vi "Calibration Main.vi"(8 "error in (no error)":errorcluster, 11 "Pump Calibration Config in":T1={"Settings"={"Cycle Period"=500.0, "Ismatech"={"VISA resource name"="", "Simulated?"=TRUE, "Pump Number"=1.0, "Reverse?"=FALSE}, "Masterflex"={"VISA resource name"="", "Simulated?"=TRUE, "Pump Number"=1.0, "Reverse?"=FALSE}, "Bronkhorst M13 Flow Meter"={"VISA resource name"="", "Simulated?"=TRUE}, "PID 2 Parameters"={"Input Device"=enum."Default", "Output Device"=enum."Default"}, "Bronkhorst M14"={"VISA resource name"="", "Simulated?"=FALSE}, "Tacmina Settings"={"Analog DAQ Task"="", "Digital DAQ Task"=""}, "KNF SIMDOS Settings"={"VISA resource name"="", "Simulated?"=TRUE}, "VICI M50 Settings"={"VISA resource name"="", "Simulated?"=TRUE, "Pump Letter"="", "Reverse?"=FALSE}, "FLOM Settings"={"VISA resource name"="", "Simulated?"=TRUE, "Pump Number"=0.0}, "Calibration Limits"={"Minimum (ml/min)"=0.0, "Maximum (ml/min)"=0.0, "Steps"=0.0}, "SSI PR Settings"={"VISA resource name"="", "Simulated?"=FALSE}}, "Flowmeter Output"=0.0, "Density"=0.0, "FL Temp"=0.0, "Speed %"=0.0, "File Refnum"=refnum, "Pump On?"=enum."Not Initialized"} {"Settings"."Masterflex"."Pump Number" min=1.0 max=20.0 step=1.0; "Settings"."Ismatech"."Pump Number" min=1.0 max=20.0 step=1.0}) -> (0 "error out":errorcluster, 3 "Pump Calibration Config out":T1={"Settings"={"Cycle Period"=500.0, "Ismatech"={"VISA resource name"="", "Simulated?"=TRUE, "Pump Number"=1.0, "Reverse?"=FALSE}, "Masterflex"={"VISA resource name"="", "Simulated?"=TRUE, "Pump Number"=1.0, "Reverse?"=FALSE}, "Bronkhorst M13 Flow Meter"={"VISA resource name"="", "Simulated?"=TRUE}, "PID 2 Parameters"={"Input Device"=enum."Default", "Output Device"=enum."Default"}, "Bronkhorst M14"={"VISA resource name"="", "Simulated?"=FALSE}, "Tacmina Settings"={"Analog DAQ Task"="", "Digital DAQ Task"=""}, "KNF SIMDOS Settings"={"VISA resource name"="", "Simulated?"=TRUE}, "VICI M50 Settings"={"VISA resource name"="", "Simulated?"=TRUE, "Pump Letter"="", "Reverse?"=FALSE}, "FLOM Settings"={"VISA resource name"="", "Simulated?"=TRUE, "Pump Number"=0.0}, "Calibration Limits"={"Minimum (ml/min)"=0.0, "Maximum (ml/min)"=0.0, "Steps"=0.0}, "SSI PR Settings"={"VISA resource name"="", "Simulated?"=FALSE}}, "Flowmeter Output"=0.0, "Density"=0.0, "FL Temp"=0.0, "Speed %"=0.0, "File Refnum"=refnum, "Pump On?"=enum."Not Initialized"} {"Settings"."Masterflex"."Pump Number" min=1.0 max=20.0 step=1.0; "Settings"."Ismatech"."Pump Number" min=1.0 max=20.0 step=1.0})   [LabVIEW 2018, in "Calibration.lvlib"]
uses:
  Pfizer Timed Seq/Software/Calibration VIs/Calibration.lvlib
  Pump Calibration Config.ctl
  Pfizer Timed Seq/Software/Ismatec ISM 831C/Controls/Ismatech Settings Cluster.ctl
  Pfizer Timed Seq/Software/Masterflex 7550-30/Controls/Settings Cluster.ctl
  Pfizer Timed Seq/Software/Bronkhorst M13 Flow Meter/Settings Cluster.ctl
  Pfizer Timed Seq/Software/Measure Instrument/PID Input Enum.ctl
  Pfizer Timed Seq/Software/Measure Instrument/PID 2 Output Enum.ctl
  Pfizer Timed Seq/Software/Mettler Toledo/Controls/Settings Cluster.ctl
  Pfizer Timed Seq/Software/Tacmina QI/Tacmina QI DAQ Setting.ctl
  Pfizer Timed Seq/Software/KNF Pump/Settings Cluster plus SIMDOS.ctl
  Pfizer Timed Seq/Software/VICI M50 Party Mode/Settings Cluster.ctl
  Pfizer Timed Seq/Software/FLOM Pump/Settings Cluster.ctl
  Pfizer Timed Seq/Software/SSI PR Class/SSI PR or LD Settings Cluster.ctl
  Pfizer Timed Seq/Software/Bronkhorst M14 Flow Meter/Settings Cluster.ctl
  Pfizer Timed Seq/Software/ASIA Pump/Pump Settings.ctl
  Pfizer Timed Seq/Software/Masterflex 75211/Masterflex 75211 DAQ Setting.ctl
  <vilib>/Platform/TimedLoop/XDataNode/timing_clust.ctl
  <vilib>/Platform/TimedLoop/XDataNode/nitl_modes.ctl
  <vilib>/Platform/TimedLoop/XDataNode/wakeup.ctl
  Pfizer Timed Seq/Software/support/Message Queue/Enqueue Message (Single).vi
  <vilib>/Utility/file.llb/Read Delimited Spreadsheet (string).vi
  <vilib>/Utility/file.llb/Write Delimited Spreadsheet (string).vi
  <vilib>/Platform/TimedLoop/XDataNode/XDataNode.xnode
  <vilib>/regexp/Match Regular Expression.xnode
  Pfizer Timed Seq/Software/KNF Pump/KNF SIMDOS.lvlib
  Pfizer Timed Seq/Software/Ismatec ISM 831C/Ismatec ISM 831C.lvlib
  Pfizer Timed Seq/Software/VICI M50 Party Mode/VICI M6 M50 Party Mode.lvlib
  Pfizer Timed Seq/Software/Masterflex 7550-30/Masterflex 7550-30.lvlib
  Pfizer Timed Seq/Software/FLOM Pump/FLOM Pump.lvlib
  Pfizer Timed Seq/Software/Bronkhorst M13 Flow Meter/Bronkhorst M13 Flow Meter.lvlib
  Pfizer Timed Seq/Software/Bronkhorst M14 Flow Meter/Bronkhorst M14 Flow Meter.lvlib
  Pfizer Timed Seq/Software/support/Message Queue/Message Queue.lvlib
  Pfizer Timed Seq/Software/SSI PR Class/SSI PR or LD Pump.lvlib
  Support/Engine.lvlib
  <vilib>/Analysis/NI_AALPro.lvlib
  <vilib>/Platform/TimedLoop/XDataNode/XDNodeRunTimeDep.lvlib
  Pfizer Timed Seq/Software/Mettler Toledo/Mettler Toledo.lvlib
  Pfizer Timed Seq/Software/Tacmina QI/Tacmina QI.lvlib
  Pfizer Timed Seq/Software/ASIA Pump.lvlib
  Pfizer Timed Seq/Software/Masterflex 75211/Masterflex 75211.lvlib
panel:
  out "Y array":dbl[](array[numeric])
  out "X array":dbl[](array[numeric])
  out "Output Selected":bool
  out "Input Selected":bool
  out "Step Array":dbl[](array[numeric])
  in  "?":enum32{"Settings", "Results"}(tab)
  in  "Settings Dialog":T16={"Cycle Period"=500.0, "Ismatech"={"VISA resource name"="", "Simulated?"=FALSE, "Pump Number"=1.0, "Reverse?"=FALSE}, "Masterflex"={"VISA resource name"="", "Simulated?"=FALSE, "Pump Number"=1.0, "Reverse?"=FALSE}, "Mettler"={"VISA resource name"="", "Simulated?"=FALSE}, "Bronkhorst M13 Flow Meter"={"VISA resource name"="", "Simulated?"=FALSE}, "Setup Parameters"={"Input Device"=enum."Default", "Output Device"=enum."Default"}, "Bronkhorst M14 Settings"={"VISA resource name"="", "Simulated?"=FALSE}, "Tacmina Settings"={"Analog DAQ Task"="", "Digital DAQ Task"=""}, "KNF SIMDOS Settings"={"VISA resource name"="", "Simulated?"=FALSE}, "ASIA Pump C"={"ASIA Pump #"=-1, "channel"=-1, "Simulated"=FALSE}, "VICI M50 Settings"={"VISA resource name"="", "Simulated?"=FALSE, "Pump Letter"="", "Reverse?"=FALSE}, "FLOM Settings"={"VISA resource name"="", "Simulated?"=FALSE, "Pump Number"=1.0}, "Calibration Limits"={"Minimum (ml/min)"=0.0, "Maximum (ml/min)"=0.0, "Steps"=0.0}, "File Name"="", "SSI PR Settings"={"VISA resource name"="", "Simulated?"=FALSE}, "Masterflex 75211 Settings"={"Analog DAQ Task"="", "Digital DAQ Task"=""}} {"Calibration Limits"."Maximum (ml/min)" max=16.5; "ASIA Pump C"."channel" min=-1 max=1 step=1; "Masterflex"."Pump Number" min=1.0 max=20.0 step=1.0; "Ismatech"."Pump Number" min=1.0 max=20.0 step=1.0}
  in  "Start Button":bool
  in  "Cancel Button":bool
  out "Y Intercept":dbl
  in  "Accept Button":bool
  in  "Decline Button":bool
  out "Calibration Graph":cluster{dbl[], dbl[]}[](graph)
  out "Calibration Slope":dbl
  out "R^2 Value":dbl format="%#.4g"
  out "Pump Status":enum16{"Off", "On", "Not Initialized"}(ring)
  # "Output Instruments"
  # "Input Instruments"
  # "Output Instruments"
  # "Input Instruments"
  # "Output Instruments"
  # "Input Instruments"
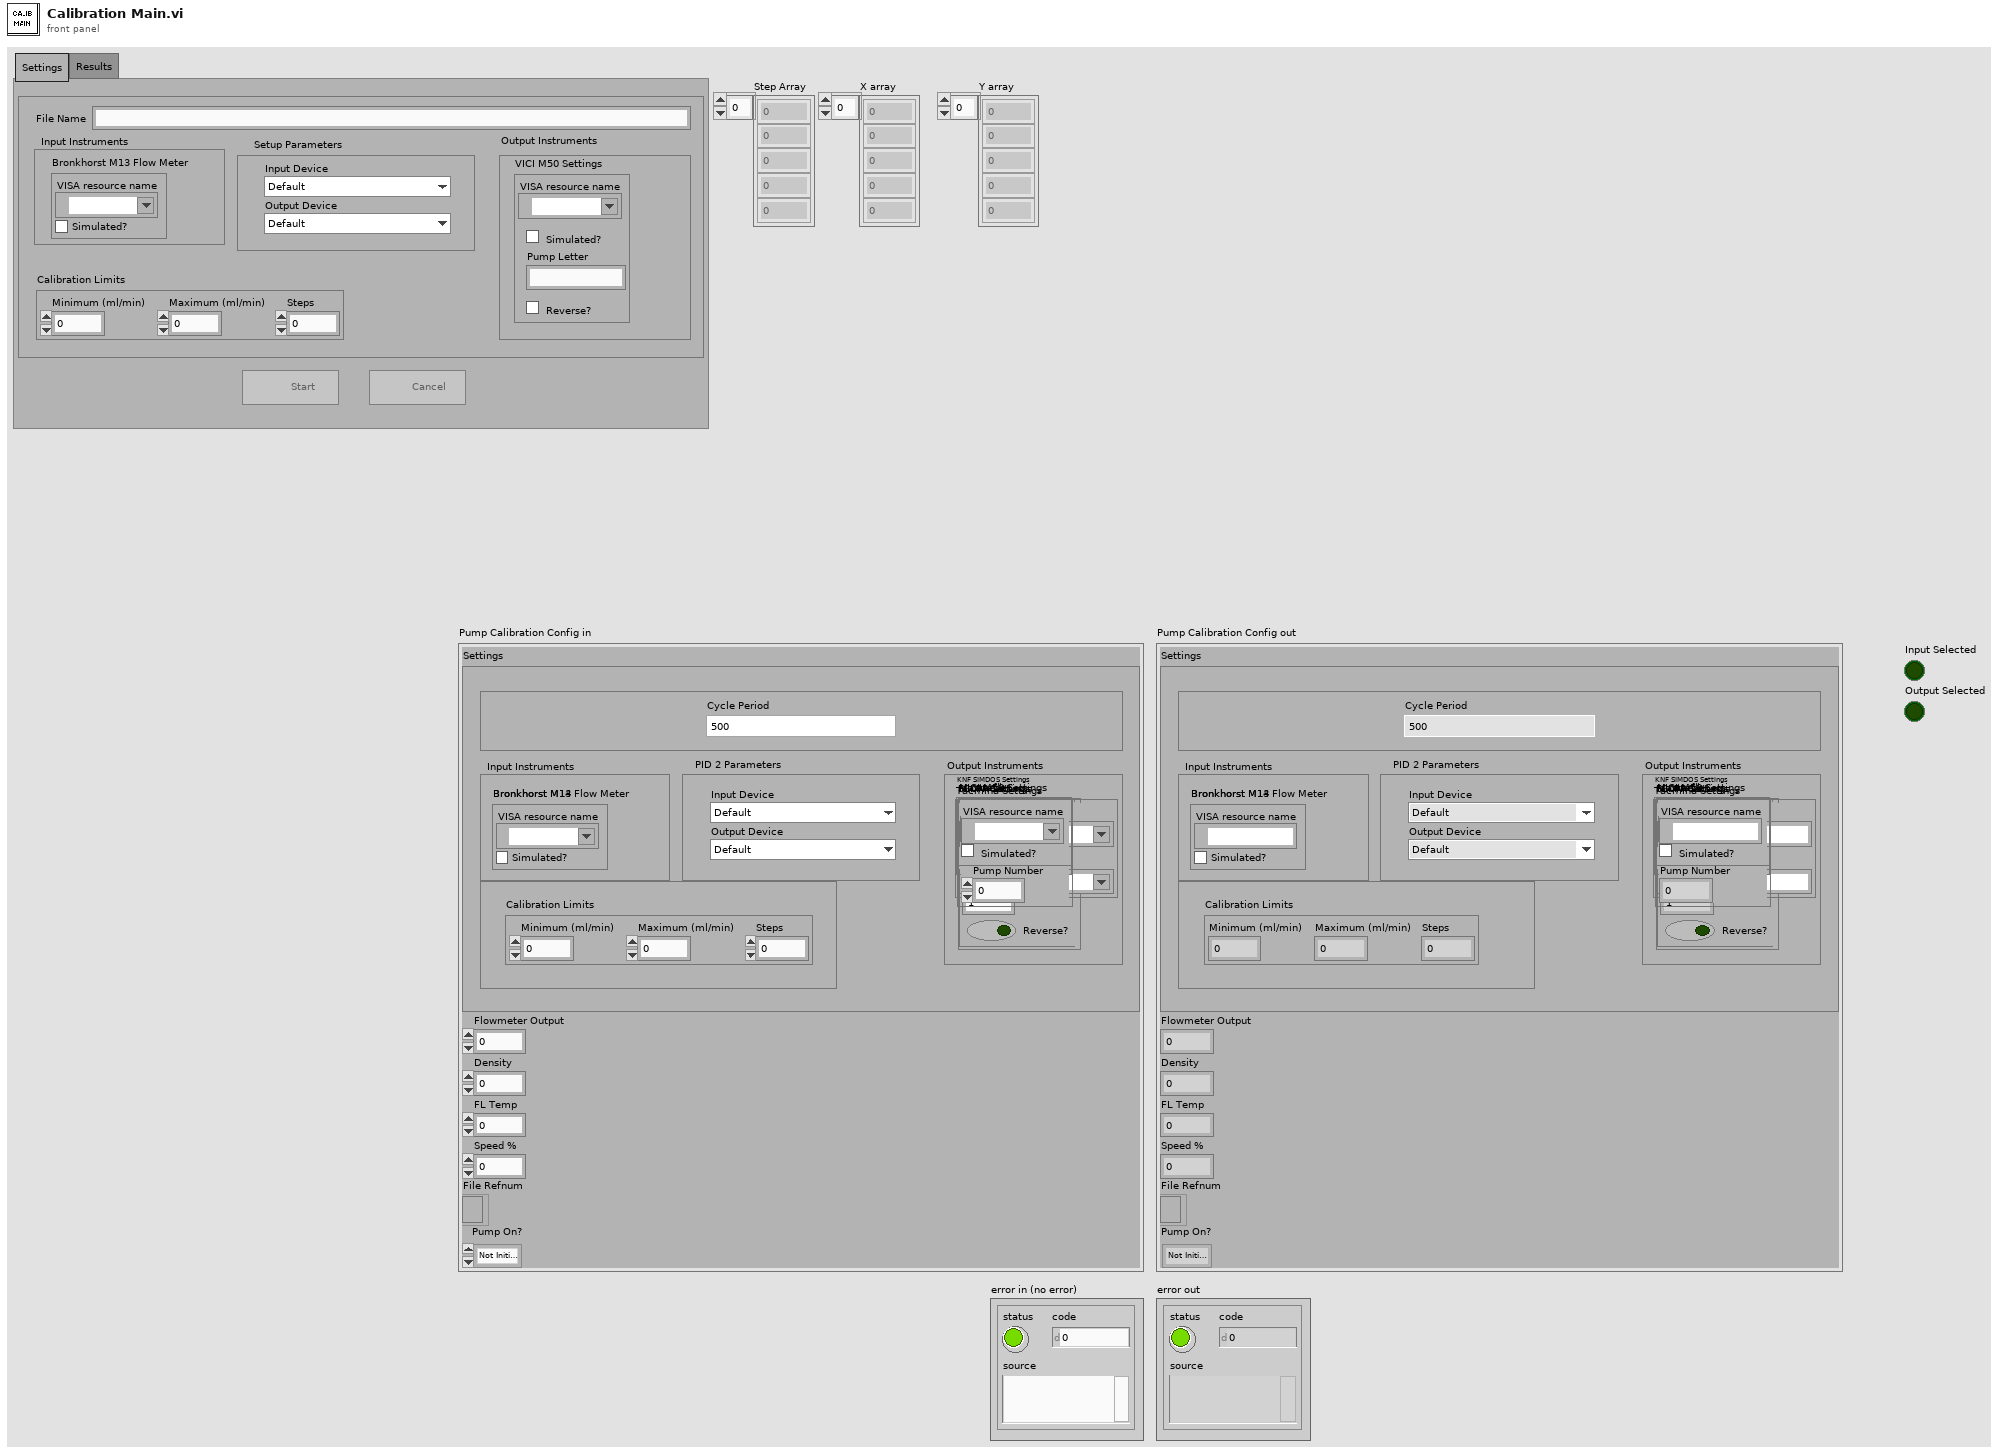
[diagram p1: front panel]
types:
  T1 = typedef "Calibration.lvlib/Pump Calibration Config.ctl" = cluster{"Settings":cluster{"Cycle Period":dbl, "Ismatech":T2, "Masterflex":T3, "Bronkhorst M13 Flow Meter":T4, "PID 2 Parameters":cluster{"Input Device":T5, "Output Device":T6}, "Bronkhorst M14":T7, "Tacmina Settings":T8, "KNF SIMDOS Settings":T9, "VICI M50 Settings":T10, "FLOM Settings":T11, "Calibration Limits":cluster{"Minimum (ml/min)":dbl, "Maximum (ml/min)":dbl, "Steps":dbl}, "SSI PR Settings":T12}, "Flowmeter Output":dbl, "Density":dbl, "FL Temp":dbl, "Speed %":dbl, "File Refnum":refnum<file>, "Pump On?":enum16{"Off", "On", "Not Initialized"}}
  T2 = typedef "Ismatec ISM 831C.lvlib/Ismatech Settings Cluster.ctl" = cluster{"VISA resource name":refnum<visa-resource-name>, "Simulated?":bool, "Pump Number":dbl, "Reverse?":bool}
  T3 = typedef "Masterflex 7550-30.lvlib/Settings Cluster.ctl" = cluster{"VISA resource name":refnum<visa-resource-name>, "Simulated?":bool, "Pump Number":dbl, "Reverse?":bool}
  T4 = typedef "Bronkhorst M13 Flow Meter.lvlib/Settings Cluster.ctl" = cluster{"VISA resource name":refnum<visa-resource-name>, "Simulated?":bool}
  T5 = typedef "PID Input Enum.ctl" = enum16{"Default", "Bronkhorst M13", "Bronkhorst M14", "Scale Rate of Change"}
  T6 = typedef "PID 2 Output Enum.ctl" = enum16{"Default", "Ismatec ISM 831C", "Masterflex 7550-30", "VICI", "Tacmina QI", "KNF SIMDOS", "ASIA Type C", "FLOM UI-22-11", "SSI PR/LD", "SSI P40", "Masterflex 75211-70"}
  T7 = typedef "Mettler Toledo.lvlib/Settings Cluster.ctl" = cluster{"VISA resource name":refnum<visa-resource-name>, "Simulated?":bool}
  T8 = typedef "Tacmina QI.lvlib/Tacmina QI DAQ Setting.ctl" = cluster{"Analog DAQ Task":refnum<k21>, "Digital DAQ Task":refnum<k21>}
  T9 = typedef "KNF SIMDOS.lvlib/Settings Cluster plus SIMDOS.ctl" = cluster{"VISA resource name":refnum<visa-resource-name>, "Simulated?":bool}
  T10 = typedef "VICI M6 M50 Party Mode.lvlib/Settings Cluster.ctl" = cluster{"VISA resource name":refnum<visa-resource-name>, "Simulated?":bool, "Pump Letter":string, "Reverse?":bool}
  T11 = typedef "FLOM Pump.lvlib/Settings Cluster.ctl" = cluster{"VISA resource name":refnum<visa-resource-name>, "Simulated?":bool, "Pump Number":dbl}
  T12 = typedef "SSI PR or LD Pump.lvlib/SSI PR or LD Settings Cluster.ctl" = cluster{"VISA resource name":refnum<visa-resource-name>, "Simulated?":bool}
  T13 = typedef "Bronkhorst M14 Flow Meter.lvlib/Settings Cluster.ctl" = cluster{"VISA resource name":refnum<visa-resource-name>, "Simulated?":bool}
  T14 = typedef "ASIA Pump.lvlib/Pump Settings.ctl" = cluster{"ASIA Pump #":i32, "channel":i32, "Simulated":bool}
  T15 = typedef "Masterflex 75211.lvlib/Masterflex 75211 DAQ Setting.ctl" = cluster{"Analog DAQ Task":refnum<k21>, "Digital DAQ Task":refnum<k21>}
  T16 = cluster{"Cycle Period":dbl, "Ismatech":T2, "Masterflex":T3, "Mettler":T7, "Bronkhorst M13 Flow Meter":T4, "Setup Parameters":cluster{"Input Device":T5, "Output Device":T6}, "Bronkhorst M14 Settings":T13, "Tacmina Settings":T8, "KNF SIMDOS Settings":T9, "ASIA Pump C":T14, "VICI M50 Settings":T10, "FLOM Settings":T11, "Calibration Limits":cluster{"Minimum (ml/min)":dbl, "Maximum (ml/min)":dbl, "Steps":dbl}, "File Name":string, "SSI PR Settings":T12, "Masterflex 75211 Settings":T15}
  T17 = enum8{"Enabled", "Disabled", "Disabled and Grayed Out"}
  T18 = cluster{"Calibration UI":refnum<queue>, "Calibration Engine":refnum<queue>}
  T19 = typedef "XDNodeRunTimeDep.lvlib/timing_clust.ctl" = cluster{"Expected End [f-1]":u64, "Actual End [f-1]":u64, "Finished Late? [f-1]":bool, "Expected End [i-1]":u64, "Actual End [i-1]":u64, "Finished Late? [i-1]":bool, "Expected Start [i]":u64, "Actual Start [i]":u64, "Expected Start [f]":u64, "Actual Start [f]":u64, "Source Name":string, "Structure Name":string, "Period":i64, "Deadline":i64, "Offset":i64, "Start":i64, "Priority":i32, "Timeout":i32, "Mode":T20, "Wakeup Reason":T21, "Error":errorcluster, "Source Type":string, "Secondary Source Type":string, "Global End Time":u64, "Global Start Time":u64, "Frame Duration":u64, "Iteration Duration":u64, "Assigned CPU":i32, "I/O Scan Engine Mode":u32}
  T20 = typedef "XDNodeRunTimeDep.lvlib/nitl_modes.ctl" = enum32{"No Change", "Process missed periods, maintain original phase", "Discard missed periods, maintain original phase", "Process missed periods, ignore original phase", "Discard missed periods, ignore original phase"}
  T21 = typedef "XDNodeRunTimeDep.lvlib/wakeup.ctl" = enum32{"Normal", "Aborted", "Asynchronous wakeup", "Timing source error", "Timed loop error", "Timeout"}
  T22 = enum16{"open", "replace", "create", "open or create", "replace or create", "replace or create with confirmation"}
  T23 = cluster{"slope min":dbl, "slope max":dbl, "intercept min":dbl, "intercept max":dbl}
  T24 = cluster{"Minimum (ml/min)":dbl, "Maximum (ml/min)":dbl, "Steps":dbl}
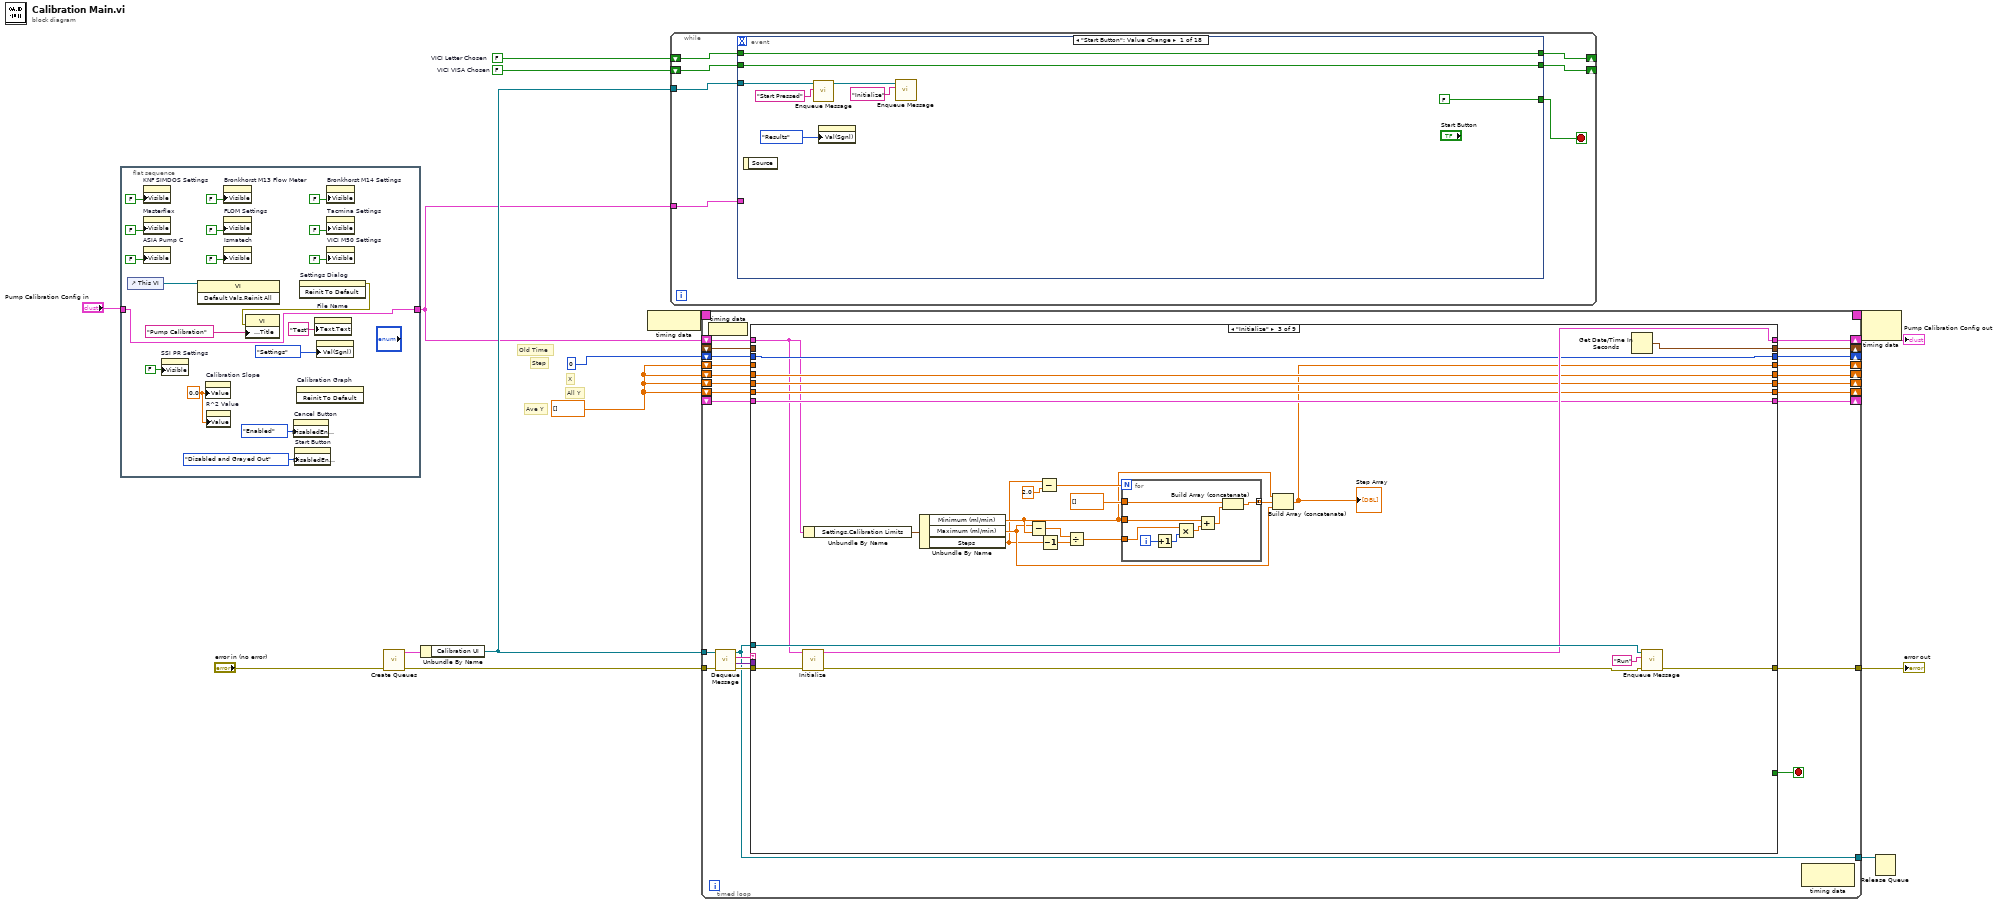
[diagram p0: block diagram]
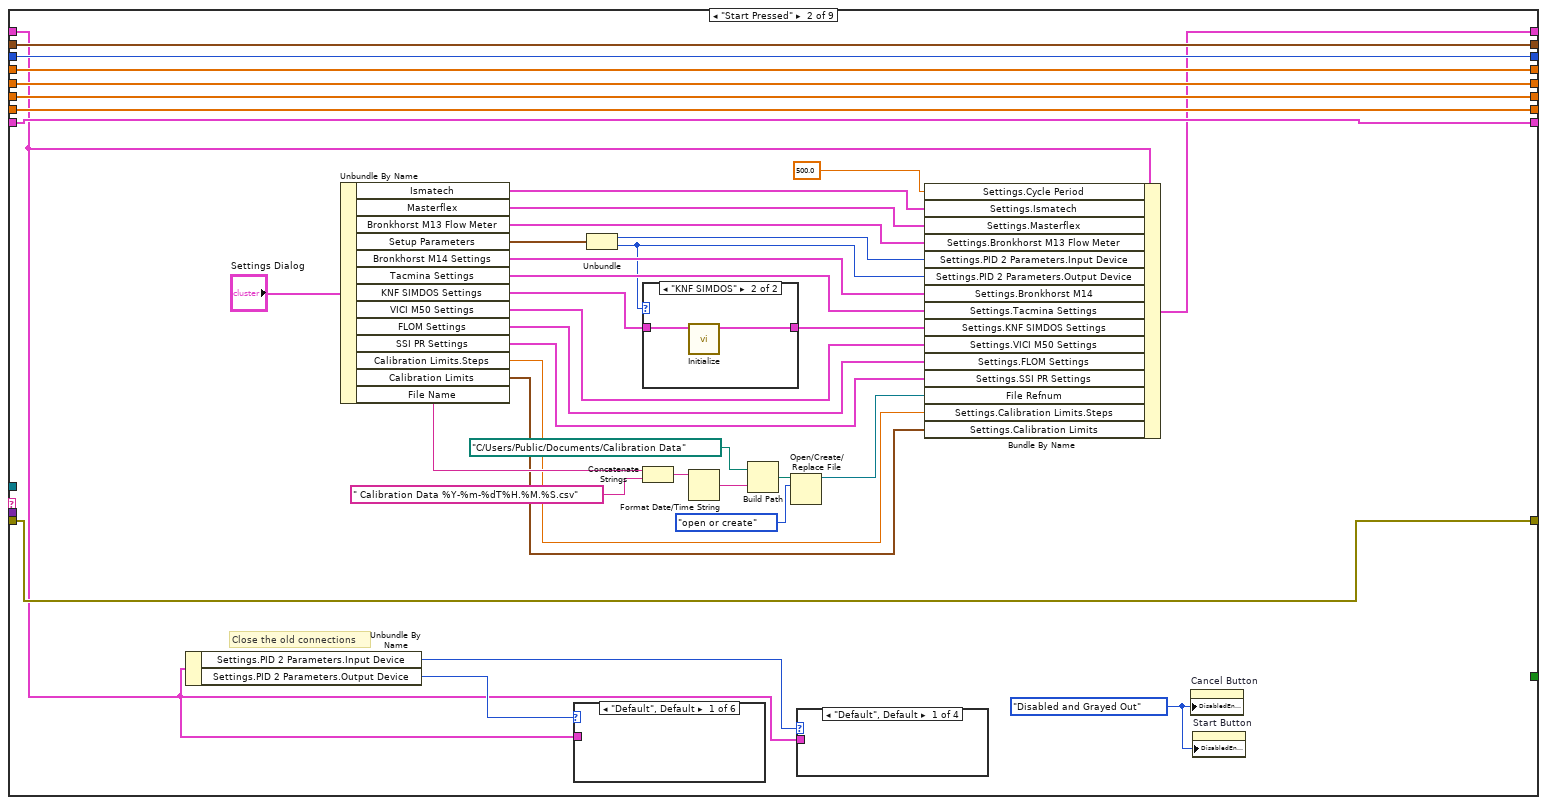
[diagram p3: hidden frame]
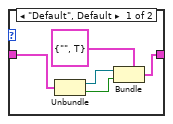
[diagram p4: hidden frame]
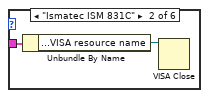
[diagram p5: hidden frame]
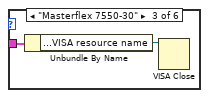
[diagram p6: hidden frame]
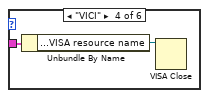
[diagram p7: hidden frame]
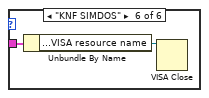
[diagram p9: hidden frame]
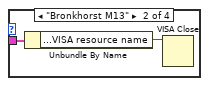
[diagram p10: hidden frame]
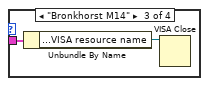
[diagram p11: hidden frame]
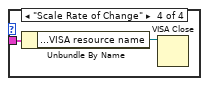
[diagram p12: hidden frame]
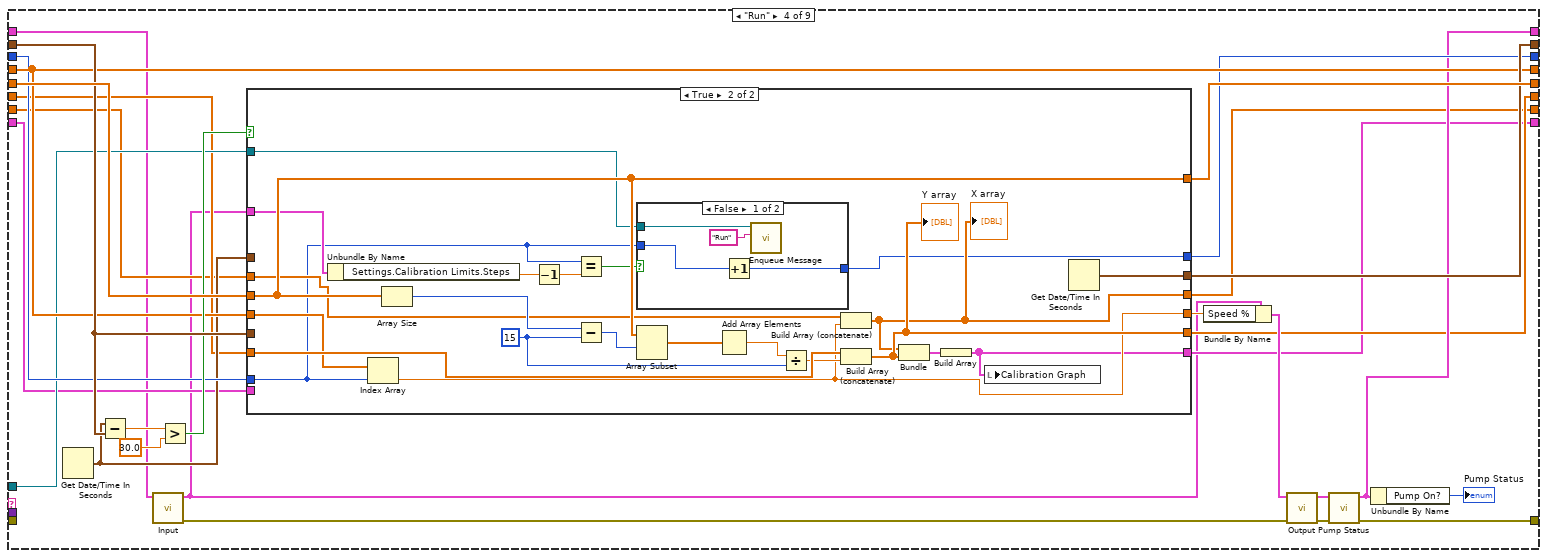
[diagram p13: hidden frame]
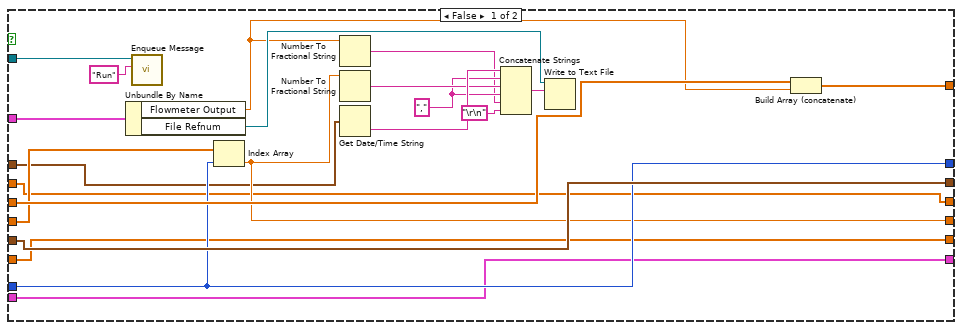
[diagram p14: hidden frame]
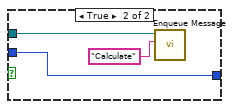
[diagram p15: hidden frame]
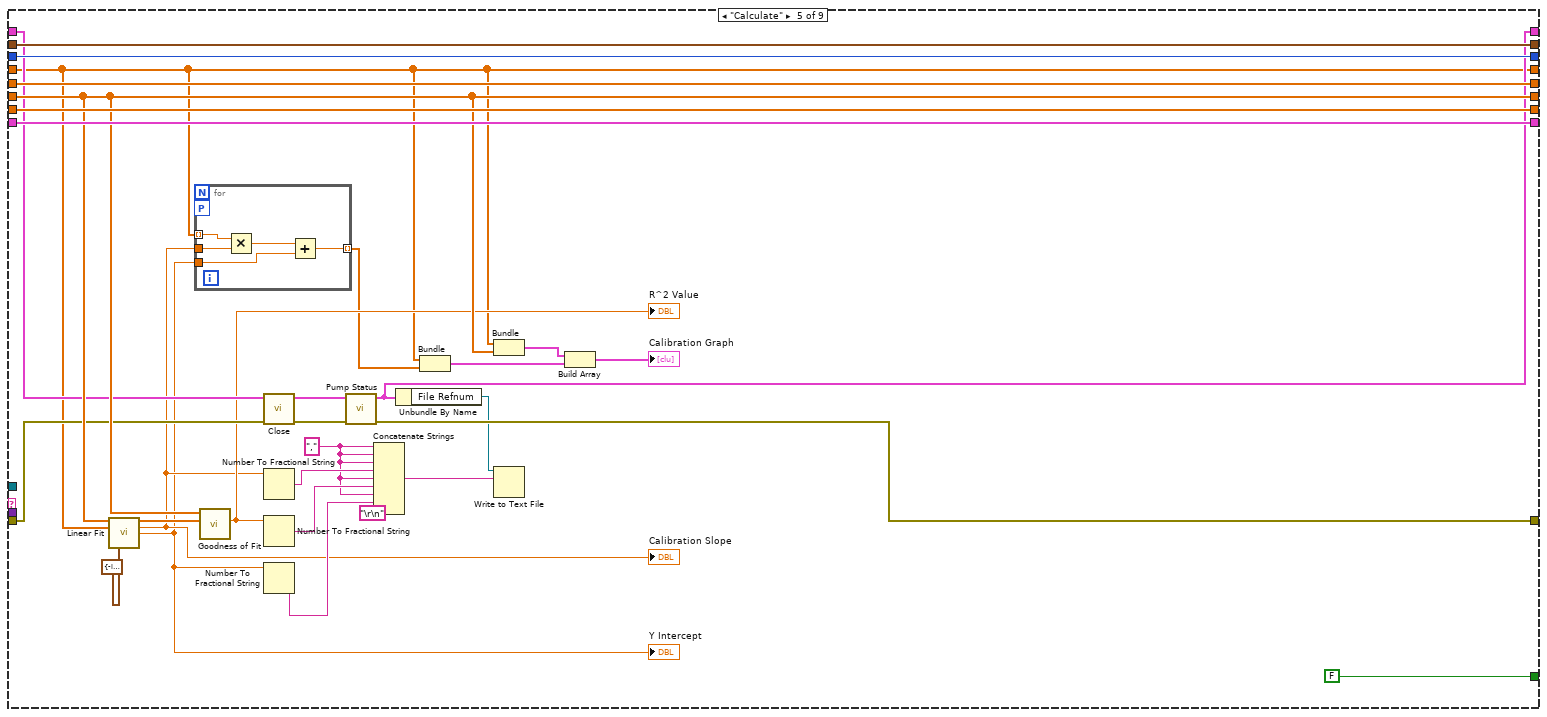
[diagram p16: hidden frame]
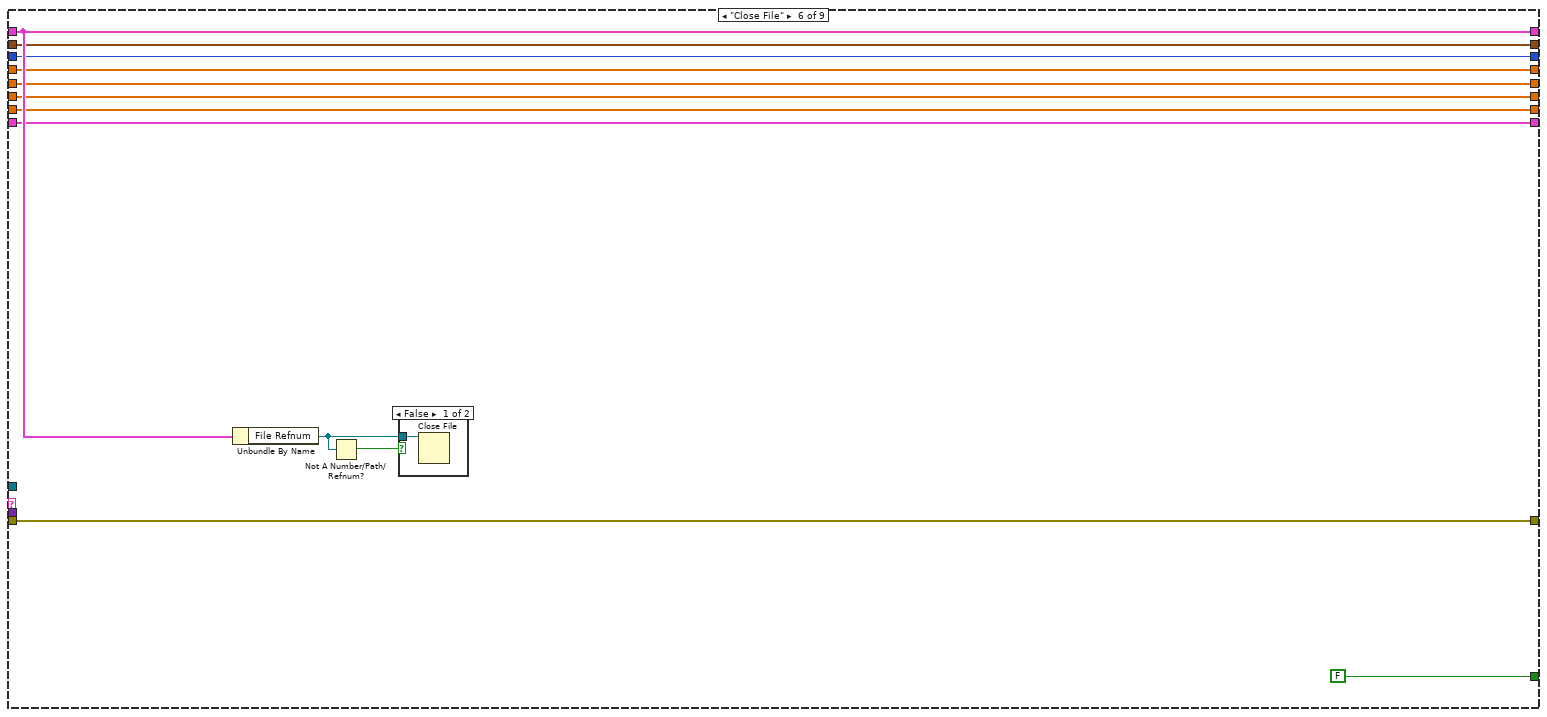
[diagram p17: hidden frame]
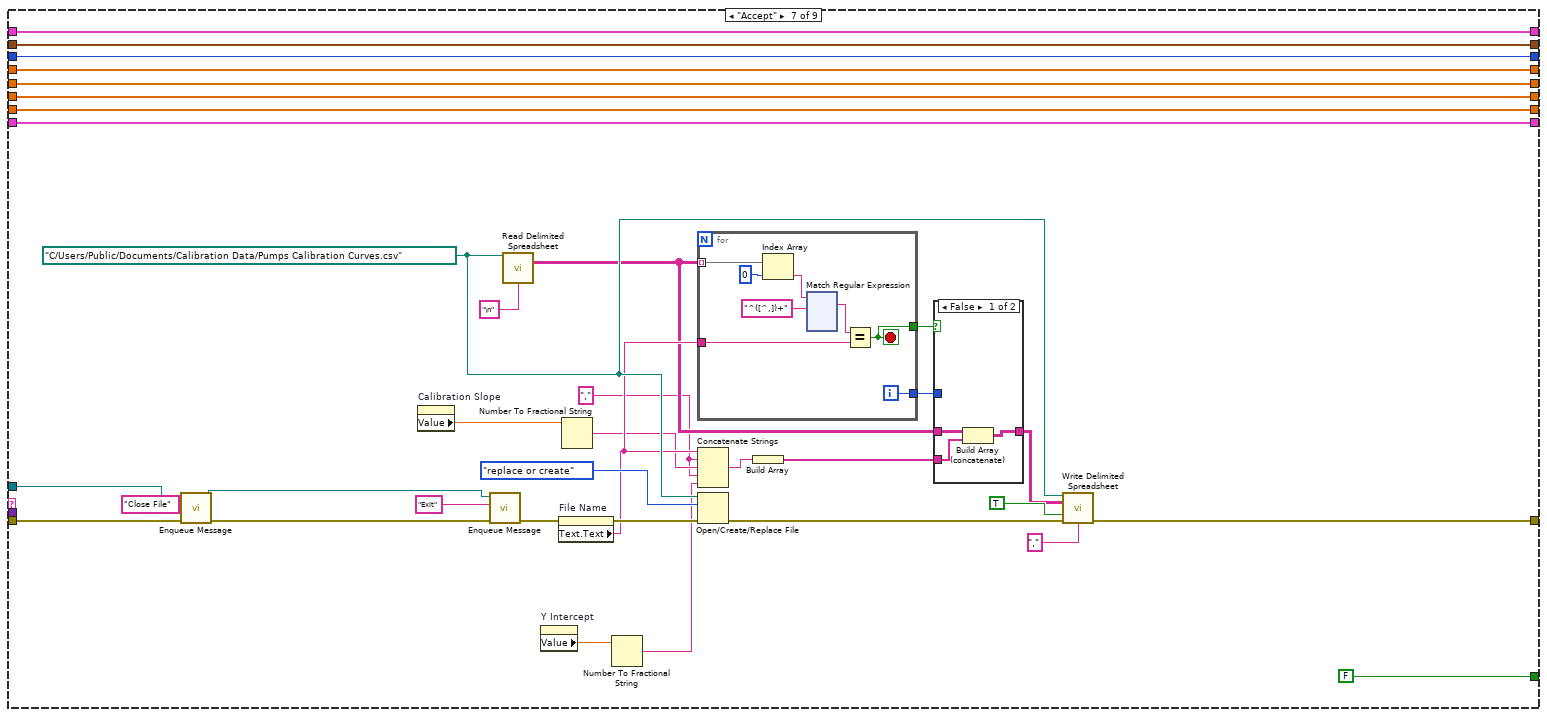
[diagram p19: hidden frame]
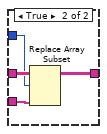
[diagram p20: hidden frame]
diagram:
  w2 = dbl[] []
  w14 = FALSE  # VICI VISA Chosen
  w15 = FALSE  # VICI Letter Chosen
  # "Old Time"
  # "Step"
  # "Ave Y"
  # "All Y"
  # "X"
  n1 = flat-sequence {
    tunnel: "Pump Calibration Config in" -> [w34]
    tunnel: [w34] -> w9
    frame #0 {
      w29 = 0.0 ("Calibration Slope")
      n2 = control-ref of="This VI"() -> (w28:refnum<vi>)
      n3 = property on="KNF SIMDOS Settings" class="Clust (strict)"("Visible"=FALSE) -> ()  [unwired: 2 in, 2 out]
      n4 = property on="Masterflex" class="Clust (strict)"("Visible"=FALSE) -> ()  [unwired: 2 in, 2 out]
      n5 = property on="ASIA Pump C" class="Clust (strict)"("Visible"=FALSE) -> ()  [unwired: 2 in, 2 out]
      n6 = property on="SSI PR Settings" class="Clust (strict)"("Visible"=FALSE) -> ()  [unwired: 2 in, 2 out]
      n7 = invoke class="VI" method="Default Vals.Reinit All"(reference=w28) -> ()  [unwired: 2 in, 3 out]
      n8 = property on="Calibration Slope" class="DigNum (strict)"("Value"=w29) -> ()  [unwired: 2 in, 2 out]
      n9 = property on="R^2 Value" class="DigNum (strict)"("Value"=w29) -> ()  [unwired: 2 in, 2 out]
      n10 = property on="Bronkhorst M13 Flow Meter" class="Clust (strict)"("Visible"=FALSE) -> ()  [unwired: 2 in, 2 out]
      n11 = property on="FLOM Settings" class="Clust (strict)"("Visible"=FALSE) -> ()  [unwired: 2 in, 2 out]
      n12 = property on="Ismatech" class="Clust (strict)"("Visible"=FALSE) -> ()  [unwired: 2 in, 2 out]
      n13 = property on="Cancel Button" class="Bool"("DisabledEnum"=T17."Enabled" ("Disabled")) -> ()  [unwired: 2 in, 2 out]
      n14 = property on="Start Button" class="Bool"("DisabledEnum"=T17."Disabled and Grayed Out" ("Disabled")) -> ()  [unwired: 2 in, 2 out]
      n15 = invoke on="Calibration Graph" class="XYGraph (strict)" method="Reinit To Default"() -> ()  [unwired: 3 in, 3 out]
      n16 = invoke on="Settings Dialog" class="Clust (strict)" method="Reinit To Default"() -> (error out=w31:errorcluster)  [unwired: 3 in, 2 out]
      n17 = property class="VI"(error in=w31, "Front Panel.Title"="Pump Calibration" ("string")) -> ()  [unwired: 1 in, 2 out]
      n18 = property on="File Name" class="Str"("Text.Text"="Test") -> ()  [unwired: 2 in, 2 out]
      n19 = property class="TabCtl (strict)"("Val(Sgnl)"=enum32{"Settings", "Results"}."Settings") -> ()  [unwired: 2 in, 2 out]
      n20 = property on="Bronkhorst M14 Settings" class="Clust (strict)"("Visible"=FALSE) -> ()  [unwired: 2 in, 2 out]
      n21 = property on="Tacmina Settings" class="Clust (strict)"("Visible"=FALSE) -> ()  [unwired: 2 in, 2 out]
      n22 = property on="VICI M50 Settings" class="Clust (strict)"("Visible"=FALSE) -> ()  [unwired: 2 in, 2 out]
    }
  }
  n23 = call "Create Queues.vi"("error in (no error)"="error in (no error)") -> ("error out"=w7:errorcluster, "Message Queues Out"=w11:T18)  [unwired: 9 in]
  n24 = Unbundle By Name(w11) -> ("Calibration UI"=w10:refnum<queue>)
  n25 = node-c288() -> (w5:T19)
  n26 = while {
    shift-right: [w40] -> _
    shift-left: w15 -> [w39]
    shift-right: [w38] -> _
    shift-left: w14 -> [w37]
    tunnel: w9 -> [w35]
    tunnel: w10 -> [w36]
    stop <- w41 stop-if-true
    n27 = event shown="[0] \"Start Button\": Value Change" {
      selector: _ -> [_ _ _ _ _ _ _ _ _ _ _ _ _ _ _ _ _ _]
      dyn-events: _ -> [_ _ _ _ _ _ _ _ _ _ _ _ _ _ _ _ _ _]
      timeout: _ -> [_ _ _ _ _ _ _ _ _ _ _ _ _ _ _ _ _ _]
      tunnel: [FALSE _ _ _ _ _ _ _ _ _ _ _ _ _ _ TRUE TRUE TRUE] -> w41
      tunnel: [w48 w51 w63 TRUE w90 w95 w108 w125 w143 w158 w169 w173 w187 w202 w221 w311 w316 w321] -> w40
      tunnel: w39 -> [w48 w51 w63 _ w90 w95 w108 w125 w143 w158 w169 w173 w187 w202 w221 w311 w316 w321]
      tunnel: [w47 w50 TRUE w78 w93 w94 w107 w124 w142 w157 w168 w172 w186 w201 w220 w310 w315 w320] -> w38
      tunnel: w37 -> [w47 w50 _ w78 w93 w94 w107 w124 w142 w157 w168 w172 w186 w201 w220 w310 w315 w320]
      tunnel: w36 -> [w43 _ _ _ _ _ _ _ _ _ _ _ _ _ _ w308 w313 w318]
      tunnel: w35 -> [_ _ _ _ _ _ _ _ _ _ _ _ _ w200 w219 _ _ _]
      event "Start Button": Value Change {
        n28 = event-data() -> ()  [unwired: 1 in, 1 out]
        n29 = call-poly "Enqueue Message.vi"("Message"="Start Pressed", "Message Queue"=w43) -> ("dup Message Queue"=w42:refnum<queue>)  [unwired: 8 in, 1 out]
        n30 = property class="TabCtl (strict)"("Val(Sgnl)"=enum32{"Settings", "Results"}."Results") -> ()  [unwired: 2 in, 2 out]
        n31 = call-poly "Enqueue Message.vi"("Message"="Initialize", "Message Queue"=w42) -> ()  [unwired: 8 in, 2 out]
      }
      event Value Change {
        n32 = event-data() -> ("OldVal"=w53:refnum<visa-resource-name>)  [unwired: 1 in]
        n33 = local read "Settings Dialog"() -> (w56:T16)
        n34 = VISA Close(VISA resource name=w53) -> (error out=w54:errorcluster)  [unwired: 1 in]
        n35 = Unbundle By Name(w56) -> ("Ismatech"=w55:T2)
        n36 = call "Initialize.vi"("error in (no error)"=w54, "Ismatech Settings"=w55) -> ("No Pump Connected"=w52:bool)  [unwired: 6 in, 3 out]
        n37 = case shown="False" w52 {
          frame False {
            n38 = local read "Input Selected"() -> (w58:bool)
            n39 = case shown="True" w58 {
              frame False {
              }
              frame True {
                n40 = control-ref of="Start Button"() -> (w60:refnum<vi>)
                n41 = property on="Property Node" class="Bool"(reference=w60, "DisabledEnum"=T17."Enabled" ("Disabled")) -> ()  [unwired: 1 in, 2 out]
              }
            }
            "Output Selected" <- TRUE ("Output Selected")
          }
          frame True {
            n42 = control-ref of="Start Button"() -> (w61:refnum<vi>)
            n43 = property on="Property Node" class="Bool"(reference=w61, "DisabledEnum"=T17."Disabled and Grayed Out" ("Disabled")) -> ()  [unwired: 1 in, 2 out]
          }
        }
      }
      event Value Change {
        n44 = event-data() -> ("OldVal"=w65:refnum<visa-resource-name>)  [unwired: 1 in]
        n45 = local read "Settings Dialog"() -> (w68:T16)
        n46 = Unbundle By Name(w68) -> ("VICI M50 Settings"=w67:T10)
        n47 = VISA Close(VISA resource name=w65) -> (error out=w66:errorcluster)  [unwired: 1 in]
        n48 = case shown="True" w63 {
          tunnel: w67 -> [_ w71]
          tunnel: w66 -> [_ w70]
          frame False {
          }
          frame True {
            n49 = call "Initialize.vi"("error in (no error)"=w70, "VICI Settings"=w71) -> ("No Pump Connected"=w69:bool)  [unwired: 6 in, 3 out]
            n50 = case shown="False" w69 {
              frame False {
                n51 = local read "Input Selected"() -> (w72:bool)
                n52 = case shown="True" w72 {
                  frame False {
                  }
                  frame True {
                    n53 = control-ref of="Start Button"() -> (w75:refnum<vi>)
                    n54 = property on="Property Node" class="Bool"(reference=w75, "DisabledEnum"=T17."Enabled" ("Disabled")) -> ()  [unwired: 1 in, 2 out]
                  }
                }
                n55 = local write "Output Selected"(TRUE) -> ()
              }
              frame True {
                n56 = control-ref of="Start Button"() -> (w76:refnum<vi>)
                n57 = property on="Property Node" class="Bool"(reference=w76, "DisabledEnum"=T17."Disabled and Grayed Out" ("Disabled")) -> ()  [unwired: 1 in, 2 out]
              }
            }
          }
        }
      }
      event Value Change {
        n58 = event-data() -> ()  [unwired: 1 in, 1 out]
        n59 = local read "Settings Dialog"() -> (w81:T16)
        n60 = Unbundle By Name(w81) -> ("VICI M50 Settings"=w80:T10)
        n61 = case shown="True" w78 {
          tunnel: w80 -> [_ w83]
          frame False {
          }
          frame True {
            n62 = call "Initialize.vi"("VICI Settings"=w83) -> ("No Pump Connected"=w82:bool)  [unwired: 7 in, 3 out]
            n63 = case shown="False" w82 {
              frame False {
                n64 = local read "Input Selected"() -> (w84:bool)
                n65 = case shown="True" w84 {
                  frame False {
                  }
                  frame True {
                    n66 = control-ref of="Start Button"() -> (w87:refnum<vi>)
                    n67 = property on="Property Node" class="Bool"(reference=w87, "DisabledEnum"=T17."Enabled" ("Disabled")) -> ()  [unwired: 1 in, 2 out]
                  }
                }
                n68 = local write "Output Selected"(TRUE) -> ()
              }
              frame True {
                n69 = control-ref of="Start Button"() -> (w88:refnum<vi>)
                n70 = property on="Property Node" class="Bool"(reference=w88, "DisabledEnum"=T17."Disabled and Grayed Out" ("Disabled")) -> ()  [unwired: 1 in, 2 out]
              }
            }
          }
        }
      }
      event Value Change {
        n71 = event-data() -> ()  [unwired: 1 in, 6 out]
        n72 = control-ref of="Start Button"() -> (w92:refnum<vi>)
        n73 = property on="Property Node" class="Bool"(reference=w92, "DisabledEnum"=T17."Enabled" ("Disabled")) -> ()  [unwired: 1 in, 2 out]
      }
      event Value Change {
        n74 = event-data() -> ("OldVal"=w97:refnum<visa-resource-name>)  [unwired: 1 in]
        n75 = local read "Settings Dialog"() -> (w99:T16)
        n76 = VISA Close(VISA resource name=w97) -> (error out=w98:errorcluster)  [unwired: 1 in]
        n77 = Unbundle By Name(w99) -> ("Masterflex"=w100:T3)
        n78 = call "Initialize.vi"("error in (no error)"=w98, "Masterflex Settings in"=w100) -> ("No Pump Connected"=w96:bool)  [unwired: 6 in, 3 out]
        n79 = case shown="False" w96 {
          frame False {
            n80 = local read "Input Selected"() -> (w101:bool)
            n81 = case shown="True" w101 {
              frame False {
              }
              frame True {
                n82 = control-ref of="Start Button"() -> (w104:refnum<vi>)
                n83 = property on="Property Node" class="Bool"(reference=w104, "DisabledEnum"=T17."Enabled" ("Disabled")) -> ()  [unwired: 1 in, 2 out]
              }
            }
            n84 = local write "Output Selected"(TRUE) -> ()
          }
          frame True {
            n85 = control-ref of="Start Button"() -> (w105:refnum<vi>)
            n86 = property on="Property Node" class="Bool"(reference=w105, "DisabledEnum"=T17."Disabled and Grayed Out" ("Disabled")) -> ()  [unwired: 1 in, 2 out]
          }
        }
      }
      event Value Change {
        n87 = event-data() -> ("OldVal"=w112:refnum<visa-resource-name>)  [unwired: 1 in]
        n88 = local read "Settings Dialog"() -> (w113:T16)
        n89 = Unbundle By Name(w113) -> ("KNF SIMDOS Settings"=w110:T9)
        n90 = VISA Close(VISA resource name=w112) -> (error out=w111:errorcluster)  [unwired: 1 in]
        n91 = call "Initialize.vi"("error in (no error)"=w111, "KNF Settings In"=w110) -> ("No Pump Connected"=w109:bool)  [unwired: 6 in, 3 out]
        n92 = case shown="False" w109 {
          frame False {
            n93 = local read "Input Selected"() -> (w114:bool)
            n94 = case shown="True" w114 {
              frame False {
              }
              frame True {
                n95 = control-ref of="Start Button"() -> (w117:refnum<vi>)
                n96 = property on="Property Node" class="Bool"(reference=w117, "DisabledEnum"=T17."Enabled" ("Disabled")) -> ()  [unwired: 1 in, 2 out]
              }
            }
            n97 = local write "Output Selected"(TRUE) -> ()
          }
          frame True {
            n98 = control-ref of="Start Button"() -> (w118:refnum<vi>)
            n99 = property on="Property Node" class="Bool"(reference=w118, "DisabledEnum"=T17."Disabled and Grayed Out" ("Disabled")) -> ()  [unwired: 1 in, 2 out]
          }
        }
      }
      event Value Change {
        n100 = event-data() -> ("OldVal"=w126:refnum<visa-resource-name>)  [unwired: 1 in]
        n101 = local read "Settings Dialog"() -> (w127:T16)
        n102 = Unbundle By Name(w127) -> ("FLOM Settings"=w121:T11)
        n103 = VISA Close(VISA resource name=w126) -> (error out=w123:errorcluster)  [unwired: 1 in]
        n104 = Unbundle By Name(w121) -> ("Pump Number"=w120:dbl)
        n105 = case shown="Default" w120 {
          tunnel: w123 -> [w130 _]
          tunnel: [w129 FALSE ("Initialized")] -> w122
          tunnel: w121 -> [w128 _]
          frame Default {
            n106 = call "Initialize.vi"("error in (no error)"=w130, "FLOM Settings in"=w128) -> ("Initialized"=w129:bool)  [unwired: 6 in, 3 out]
          }
          frame 0 {
            n107 = One Button Dialog(message="Choose a Pump Number") -> ()  [unwired: 1 in, 1 out]
          }
        }
        n108 = case shown="True" w122 {
          frame False {
            n109 = control-ref of="Start Button"() -> (w133:refnum<vi>)
            n110 = property on="Property Node" class="Bool"(reference=w133, "DisabledEnum"=T17."Disabled and Grayed Out" ("Disabled")) -> ()  [unwired: 1 in, 2 out]
          }
          frame True {
            n111 = local read "Input Selected"() -> (w135:bool)
            n112 = case shown="True" w135 {
              frame False {
              }
              frame True {
                n113 = control-ref of="Start Button"() -> (w138:refnum<vi>)
                n114 = property on="Property Node" class="Bool"(reference=w138, "DisabledEnum"=T17."Enabled" ("Disabled")) -> ()  [unwired: 1 in, 2 out]
              }
            }
            n115 = local write "Output Selected"(TRUE) -> ()
          }
        }
      }
      event Value Change {
        n116 = event-data() -> ()  [unwired: 1 in, 1 out]
        n117 = local read "Settings Dialog"() -> (w144:T16)
        n118 = Unbundle By Name(w144) -> ("FLOM Settings"=w140:T11)
        n119 = Unbundle By Name(w140) -> ("Pump Number"=w139:dbl)
        n120 = case shown="Default" w139 {
          tunnel: [w146 FALSE ("Initialized")] -> w141
          tunnel: w140 -> [w145 _]
          frame Default {
            n121 = call "Initialize.vi"("FLOM Settings in"=w145) -> ("Initialized"=w146:bool)  [unwired: 7 in, 3 out]
          }
          frame 0 {
            n122 = One Button Dialog(message="Choose a non-zero Pump Number") -> ()  [unwired: 1 in, 1 out]
          }
        }
        n123 = case shown="True" w141 {
          frame False {
            n124 = control-ref of="Start Button"() -> (w149:refnum<vi>)
            n125 = property on="Property Node" class="Bool"(reference=w149, "DisabledEnum"=T17."Disabled and Grayed Out" ("Disabled")) -> ()  [unwired: 1 in, 2 out]
          }
          frame True {
            n126 = local read "Input Selected"() -> (w151:bool)
            n127 = case shown="True" w151 {
              frame False {
              }
              frame True {
                n128 = control-ref of="Start Button"() -> (w154:refnum<vi>)
                n129 = property on="Property Node" class="Bool"(reference=w154, "DisabledEnum"=T17."Enabled" ("Disabled")) -> ()  [unwired: 1 in, 2 out]
              }
            }
            n130 = local write "Output Selected"(TRUE) -> ()
          }
        }
      }
      event Value Change {
        n131 = event-data() -> ()  [unwired: 1 in, 1 out]
        n132 = local read "Settings Dialog"() -> (w159:T16)
        n133 = Unbundle By Name(w159) -> ("SSI PR Settings"=w155:T12)
        n134 = call "Initialize.vi"("SSI PR Settings In"=w155) -> ("Initialized"=w156:bool)  [unwired: 7 in, 3 out]
        n135 = case shown="True" w156 {
          frame False {
            n136 = control-ref of="Start Button"() -> (w160:refnum<vi>)
            n137 = property on="Property Node" class="Bool"(reference=w160, "DisabledEnum"=T17."Disabled and Grayed Out" ("Disabled")) -> ()  [unwired: 1 in, 2 out]
          }
          frame True {
            n138 = local read "Input Selected"() -> (w162:bool)
            n139 = case shown="True" w162 {
              frame False {
              }
              frame True {
                n140 = control-ref of="Start Button"() -> (w165:refnum<vi>)
                n141 = property on="Property Node" class="Bool"(reference=w165, "DisabledEnum"=T17."Enabled" ("Disabled")) -> ()  [unwired: 1 in, 2 out]
              }
            }
            n142 = local write "Output Selected"(TRUE) -> ()
          }
        }
      }
      event Value Change {
        n143 = event-data() -> ()  [unwired: 1 in, 6 out]
        n144 = local read "Input Selected"() -> (w166:bool)
        n145 = case shown="True" w166 {
          frame False {
          }
          frame True {
            n146 = control-ref of="Start Button"() -> (w171:refnum<vi>)
            n147 = property on="Property Node" class="Bool"(reference=w171, "DisabledEnum"=T17."Enabled" ("Disabled")) -> ()  [unwired: 1 in, 2 out]
          }
        }
        n148 = local write "Output Selected"(TRUE) -> ()
      }
      event Value Change {
        n149 = event-data() -> ("OldVal"=w175:refnum<visa-resource-name>)  [unwired: 1 in]
        n150 = local read "Settings Dialog"() -> (w178:T16)
        n151 = Unbundle By Name(w178) -> ("Bronkhorst M13 Flow Meter"=w177:T4)
        n152 = VISA Close(VISA resource name=w175) -> (error out=w176:errorcluster)  [unwired: 1 in]
        n153 = call "Initialize.vi"("error in (no error)"=w176, "Bronkhorst Settings in"=w177) -> ("No Meter Connnected"=w174:bool)  [unwired: 7 in, 2 out]
        n154 = case shown="False" w174 {
          frame False {
            n155 = local read "Output Selected"() -> (w179:bool)
            n156 = case shown="True" w179 {
              frame False {
              }
              frame True {
                n157 = control-ref of="Start Button"() -> (w182:refnum<vi>)
                n158 = property on="Property Node" class="Bool"(reference=w182, "DisabledEnum"=T17."Enabled" ("Disabled")) -> ()  [unwired: 1 in, 2 out]
              }
            }
            "Input Selected" <- TRUE ("Input Selected")
          }
          frame True {
            n159 = control-ref of="Start Button"() -> (w184:refnum<vi>)
            n160 = property on="Property Node" class="Bool"(reference=w184, "DisabledEnum"=T17."Disabled and Grayed Out" ("Disabled")) -> ()  [unwired: 1 in, 2 out]
            n161 = local write "Input Selected"(FALSE ("Input Selected")) -> ()
          }
        }
      }
      event Value Change {
        n162 = event-data() -> ("OldVal"=w189:refnum<visa-resource-name>)  [unwired: 1 in]
        n163 = local read "Settings Dialog"() -> (w192:T16)
        n164 = Unbundle By Name(w192) -> ("Bronkhorst M14 Settings"=w191:T13)
        n165 = VISA Close(VISA resource name=w189) -> (error out=w190:errorcluster)  [unwired: 1 in]
        n166 = call "Initialize.vi"("error in (no error)"=w190, "Bronkhorst Settings in"=w191) -> ("No Meter Connected"=w188:bool)  [unwired: 7 in, 2 out]
        n167 = case shown="False" w188 {
          frame False {
            n168 = local read "Output Selected"() -> (w193:bool)
            n169 = case shown="True" w193 {
              frame False {
              }
              frame True {
                n170 = control-ref of="Start Button"() -> (w196:refnum<vi>)
                n171 = property on="Property Node" class="Bool"(reference=w196, "DisabledEnum"=T17."Enabled" ("Disabled")) -> ()  [unwired: 1 in, 2 out]
              }
            }
            n172 = local write "Input Selected"(TRUE ("Input Selected")) -> ()
          }
          frame True {
            n173 = property on="Start Button" class="Bool"("DisabledEnum"=T17."Disabled and Grayed Out" ("Disabled")) -> ()  [unwired: 2 in, 2 out]
            n174 = local write "Input Selected"(FALSE ("Input Selected")) -> ()
          }
        }
      }
      event Value Change {
        n175 = event-data() -> ("NewVal"=w203:T5)  [unwired: 1 in]
        n176 = case "Show the correct settings" shown="\"Bronkhorst M13\"" w203 {
          tunnel: w200 -> [w205 w211 _]
          tunnel: [16.5 ("Data Entry Limits:Maximum") 166.0 ("Data Entry Limits:Maximum") inf] -> w199
          frame "Bronkhorst M13" {
            n177 = Unbundle By Name(w205) -> ("Settings.Bronkhorst M13 Flow Meter.VISA resource name"=w207:refnum<visa-resource-name>)
            n178 = control-ref of="VISA resource name"() -> (w208:refnum<vi>)
            n179 = property on="Bronkhorst M14 Settings" class="Clust (strict)"("Visible"=FALSE) -> ()  [unwired: 2 in, 2 out]
            n180 = property on="Bronkhorst M13 Flow Meter" class="Clust (strict)"("Visible"=TRUE) -> ()  [unwired: 2 in, 2 out]
            n181 = property on="Property Node" class="VISAName"(reference=w208, "Value"=w207) -> ()  [unwired: 1 in, 2 out]
          }
          frame "Bronkhorst M14" {
            n182 = Unbundle By Name(w211) -> ("Settings.Bronkhorst M14.VISA resource name"=w213:refnum<visa-resource-name>)
            n183 = control-ref of="VISA resource name"() -> (w214:refnum<vi>)
            n184 = property on="Bronkhorst M14 Settings" class="Clust (strict)"("Visible"=TRUE) -> ()  [unwired: 2 in, 2 out]
            n185 = property on="Bronkhorst M13 Flow Meter" class="Clust (strict)"("Visible"=FALSE) -> ()  [unwired: 2 in, 2 out]
            n186 = property on="Property Node" class="VISAName"(reference=w214, "Value"=w213) -> ()  [unwired: 1 in, 2 out]
          }
          frame "Default", Default {
            n187 = property on="Bronkhorst M14 Settings" class="Clust (strict)"("Visible"=FALSE) -> ()  [unwired: 2 in, 2 out]
            n188 = property on="Bronkhorst M13 Flow Meter" class="Clust (strict)"("Visible"=FALSE) -> ()  [unwired: 2 in, 2 out]
          }
        }
        n189 = property on="Maximum (ml/min)" class="DigNum (strict)"("Maximum"=w199) -> ()  [unwired: 2 in, 2 out]
      }
      event Value Change {
        n190 = event-data() -> ("NewVal"=w222:T6)  [unwired: 1 in]
        n191 = case "Show the correct settings" shown="\"Masterflex 75211-70\"" w222 {
          tunnel: w219 -> [w229 w240 w251 w263 _ _ _ w295 _]
          frame "Ismatec ISM 831C" {
            n192 = Unbundle By Name(w229) -> ("Settings.Ismatech.VISA resource name"=w230:refnum<visa-resource-name>)
            n193 = property on="VICI M50 Settings" class="Clust (strict)"("Visible"=FALSE) -> ()  [unwired: 2 in, 2 out]
            n194 = property on="Masterflex" class="Clust (strict)"("Visible"=FALSE) -> ()  [unwired: 2 in, 2 out]
            n195 = control-ref of="VISA resource name"() -> (w231:refnum<vi>)
            n196 = property on="Ismatech" class="Clust (strict)"("Visible"=TRUE) -> ()  [unwired: 2 in, 2 out]
            n197 = property on="FLOM Settings" class="Clust (strict)"("Visible"=FALSE) -> ()  [unwired: 2 in, 2 out]
            n198 = property on="Property Node" class="VISAName"(reference=w231, "Value"=w230) -> ()  [unwired: 1 in, 2 out]
            n199 = property on="KNF SIMDOS Settings" class="Clust (strict)"("Visible"=FALSE) -> ()  [unwired: 2 in, 2 out]
            n200 = property on="Tacmina Settings" class="Clust (strict)"("Visible"=FALSE) -> ()  [unwired: 2 in, 2 out]
            n201 = property on="Masterflex 75211 Settings" class="Clust (strict)"("Visible"=FALSE) -> ()  [unwired: 2 in, 2 out]
            n202 = property on="SSI PR Settings" class="Clust (strict)"("Visible"=FALSE) -> ()  [unwired: 2 in, 2 out]
          }
          frame "FLOM UI-22-11" {
            n203 = Unbundle By Name(w240) -> ("Settings.FLOM Settings.VISA resource name"=w241:refnum<visa-resource-name>)
            n204 = property on="Ismatech" class="Clust (strict)"("Visible"=FALSE) -> ()  [unwired: 2 in, 2 out]
            n205 = property on="FLOM Settings" class="Clust (strict)"("Visible"=TRUE) -> ()  [unwired: 2 in, 2 out]
            n206 = property on="VICI M50 Settings" class="Clust (strict)"("Visible"=FALSE) -> ()  [unwired: 2 in, 2 out]
            n207 = property on="Masterflex" class="Clust (strict)"("Visible"=FALSE) -> ()  [unwired: 2 in, 2 out]
            n208 = control-ref of="VISA resource name"() -> (w242:refnum<vi>)
            n209 = property on="Property Node" class="VISAName"(reference=w242, "Value"=w241) -> ()  [unwired: 1 in, 2 out]
            n210 = property on="Tacmina Settings" class="Clust (strict)"("Visible"=FALSE) -> ()  [unwired: 2 in, 2 out]
            n211 = property on="KNF SIMDOS Settings" class="Clust (strict)"("Visible"=FALSE) -> ()  [unwired: 2 in, 2 out]
            n212 = property on="Masterflex 75211 Settings" class="Clust (strict)"("Visible"=FALSE) -> ()  [unwired: 2 in, 2 out]
            n213 = property on="SSI PR Settings" class="Clust (strict)"("Visible"=FALSE) -> ()  [unwired: 2 in, 2 out]
          }
          frame "Masterflex 7550-30" {
            n214 = Unbundle By Name(w251) -> ("Settings.Masterflex.VISA resource name"=w252:refnum<visa-resource-name>)
            n215 = property on="Ismatech" class="Clust (strict)"("Visible"=FALSE) -> ()  [unwired: 2 in, 2 out]
            n216 = property on="FLOM Settings" class="Clust (strict)"("Visible"=FALSE) -> ()  [unwired: 2 in, 2 out]
            n217 = property on="VICI M50 Settings" class="Clust (strict)"("Visible"=FALSE) -> ()  [unwired: 2 in, 2 out]
            n218 = property on="Masterflex" class="Clust (strict)"("Visible"=TRUE) -> ()  [unwired: 2 in, 2 out]
            n219 = control-ref of="VISA resource name"() -> (w253:refnum<vi>)
            n220 = property on="Tacmina Settings" class="Clust (strict)"("Visible"=FALSE) -> ()  [unwired: 2 in, 2 out]
            n221 = property on="KNF SIMDOS Settings" class="Clust (strict)"("Visible"=FALSE) -> ()  [unwired: 2 in, 2 out]
            n222 = property on="Property Node" class="VISAName"(reference=w253, "Value"=w252) -> ()  [unwired: 1 in, 2 out]
            n223 = property on="Masterflex 75211 Settings" class="Clust (strict)"("Visible"=FALSE) -> ()  [unwired: 2 in, 2 out]
            n224 = property on="SSI PR Settings" class="Clust (strict)"("Visible"=FALSE) -> ()  [unwired: 2 in, 2 out]
          }
          frame "VICI" {
            n225 = property on="Ismatech" class="Clust (strict)"("Visible"=FALSE) -> ()  [unwired: 2 in, 2 out]
            n226 = property on="FLOM Settings" class="Clust (strict)"("Visible"=FALSE) -> ()  [unwired: 2 in, 2 out]
            n227 = Unbundle By Name(w263) -> ("Settings.VICI M50 Settings.VISA resource name"=w262:refnum<visa-resource-name>)
            n228 = property on="VICI M50 Settings" class="Clust (strict)"("Visible"=TRUE) -> ()  [unwired: 2 in, 2 out]
            n229 = property on="Masterflex" class="Clust (strict)"("Visible"=FALSE) -> ()  [unwired: 2 in, 2 out]
            n230 = property on="KNF SIMDOS Settings" class="Clust (strict)"("Visible"=FALSE) -> ()  [unwired: 2 in, 2 out]
            n231 = property on="Tacmina Settings" class="Clust (strict)"("Visible"=FALSE) -> ()  [unwired: 2 in, 2 out]
            n232 = property on="VISA resource name" class="VISAName"("Value"=w262) -> ()  [unwired: 2 in, 2 out]
            n233 = property on="Masterflex 75211 Settings" class="Clust (strict)"("Visible"=FALSE) -> ()  [unwired: 2 in, 2 out]
            n234 = property on="SSI PR Settings" class="Clust (strict)"("Visible"=FALSE) -> ()  [unwired: 2 in, 2 out]
          }
          frame "Default", Default {
            n235 = property on="KNF SIMDOS Settings" class="Clust (strict)"("Visible"=FALSE) -> ()  [unwired: 2 in, 2 out]
            n236 = property on="FLOM Settings" class="Clust (strict)"("Visible"=FALSE) -> ()  [unwired: 2 in, 2 out]
            n237 = property on="Masterflex" class="Clust (strict)"("Visible"=FALSE) -> ()  [unwired: 2 in, 2 out]
            n238 = property on="Tacmina Settings" class="Clust (strict)"("Visible"=FALSE) -> ()  [unwired: 2 in, 2 out]
            n239 = property on="VICI M50 Settings" class="Clust (strict)"("Visible"=FALSE) -> ()  [unwired: 2 in, 2 out]
            n240 = property on="Ismatech" class="Clust (strict)"("Visible"=FALSE) -> ()  [unwired: 2 in, 2 out]
            n241 = property on="Masterflex 75211 Settings" class="Clust (strict)"("Visible"=FALSE) -> ()  [unwired: 2 in, 2 out]
            n242 = property on="SSI PR Settings" class="Clust (strict)"("Visible"=FALSE) -> ()  [unwired: 2 in, 2 out]
          }
          frame "Tacmina QI" {
            n243 = property on="FLOM Settings" class="Clust (strict)"("Visible"=FALSE) -> ()  [unwired: 2 in, 2 out]
            n244 = property on="KNF SIMDOS Settings" class="Clust (strict)"("Visible"=FALSE) -> ()  [unwired: 2 in, 2 out]
            n245 = property on="Tacmina Settings" class="Clust (strict)"("Visible"=TRUE) -> ()  [unwired: 2 in, 2 out]
            n246 = property on="Ismatech" class="Clust (strict)"("Visible"=FALSE) -> ()  [unwired: 2 in, 2 out]
            n247 = property on="Masterflex" class="Clust (strict)"("Visible"=FALSE) -> ()  [unwired: 2 in, 2 out]
            n248 = property on="VICI M50 Settings" class="Clust (strict)"("Visible"=FALSE) -> ()  [unwired: 2 in, 2 out]
            n249 = property on="Masterflex 75211 Settings" class="Clust (strict)"("Visible"=FALSE) -> ()  [unwired: 2 in, 2 out]
            n250 = property on="SSI PR Settings" class="Clust (strict)"("Visible"=FALSE) -> ()  [unwired: 2 in, 2 out]
          }
          frame "SSI PR/LD" {
            n251 = property on="FLOM Settings" class="Clust (strict)"("Visible"=FALSE) -> ()  [unwired: 2 in, 2 out]
            n252 = property on="KNF SIMDOS Settings" class="Clust (strict)"("Visible"=FALSE) -> ()  [unwired: 2 in, 2 out]
            n253 = property on="Tacmina Settings" class="Clust (strict)"("Visible"=FALSE) -> ()  [unwired: 2 in, 2 out]
            n254 = property on="Ismatech" class="Clust (strict)"("Visible"=FALSE) -> ()  [unwired: 2 in, 2 out]
            n255 = property on="Masterflex" class="Clust (strict)"("Visible"=FALSE) -> ()  [unwired: 2 in, 2 out]
            n256 = property on="VICI M50 Settings" class="Clust (strict)"("Visible"=FALSE) -> ()  [unwired: 2 in, 2 out]
            n257 = property on="Masterflex 75211 Settings" class="Clust (strict)"("Visible"=FALSE) -> ()  [unwired: 2 in, 2 out]
            n258 = property on="SSI PR Settings" class="Clust (strict)"("Visible"=TRUE) -> ()  [unwired: 2 in, 2 out]
          }
          frame "KNF SIMDOS" {
            n259 = property on="Ismatech" class="Clust (strict)"("Visible"=FALSE) -> ()  [unwired: 2 in, 2 out]
            n260 = property on="FLOM Settings" class="Clust (strict)"("Visible"=FALSE) -> ()  [unwired: 2 in, 2 out]
            n261 = Unbundle By Name(w295) -> ("Settings.KNF SIMDOS Settings.VISA resource name"=w296:refnum<visa-resource-name>)
            n262 = property on="VICI M50 Settings" class="Clust (strict)"("Visible"=FALSE) -> ()  [unwired: 2 in, 2 out]
            n263 = property on="Masterflex" class="Clust (strict)"("Visible"=FALSE) -> ()  [unwired: 2 in, 2 out]
            n264 = property on="Tacmina Settings" class="Clust (strict)"("Visible"=FALSE) -> ()  [unwired: 2 in, 2 out]
            n265 = property on="KNF SIMDOS Settings" class="Clust (strict)"("Visible"=TRUE) -> ()  [unwired: 2 in, 2 out]
            n266 = property on="VISA resource name" class="VISAName"("Value"=w296) -> ()  [unwired: 2 in, 2 out]
            n267 = property on="Masterflex 75211 Settings" class="Clust (strict)"("Visible"=FALSE) -> ()  [unwired: 2 in, 2 out]
            n268 = property on="SSI PR Settings" class="Clust (strict)"("Visible"=FALSE) -> ()  [unwired: 2 in, 2 out]
          }
          frame "Masterflex 75211-70" {
            n269 = property on="FLOM Settings" class="Clust (strict)"("Visible"=FALSE) -> ()  [unwired: 2 in, 2 out]
            n270 = property on="KNF SIMDOS Settings" class="Clust (strict)"("Visible"=FALSE) -> ()  [unwired: 2 in, 2 out]
            n271 = property on="Tacmina Settings" class="Clust (strict)"("Visible"=FALSE) -> ()  [unwired: 2 in, 2 out]
            n272 = property on="Ismatech" class="Clust (strict)"("Visible"=FALSE) -> ()  [unwired: 2 in, 2 out]
            n273 = property on="Masterflex" class="Clust (strict)"("Visible"=FALSE) -> ()  [unwired: 2 in, 2 out]
            n274 = property on="VICI M50 Settings" class="Clust (strict)"("Visible"=FALSE) -> ()  [unwired: 2 in, 2 out]
            n275 = property on="Masterflex 75211 Settings" class="Clust (strict)"("Visible"=TRUE) -> ()  [unwired: 2 in, 2 out]
            n276 = property on="SSI PR Settings" class="Clust (strict)"("Visible"=FALSE) -> ()  [unwired: 2 in, 2 out]
          }
        }
      }
      event "Cancel Button": Value Change; Panel Close {
        # "True: Stop While Loop and Close Dialog"
        n277 = event-data() -> ()  [unwired: 1 in, 1 out]
        n278 = call-poly "Enqueue Message.vi"("Message"="Exit", "Message Queue"=w308) -> ()  [unwired: 8 in, 2 out]
      }
      event "Accept Button": Value Change {
        # "True: Stop While Loop and Close Dialog"
        n279 = event-data() -> ()  [unwired: 1 in, 1 out]
        n280 = call-poly "Enqueue Message.vi"("Message"="Accept", "Message Queue"=w313) -> ()  [unwired: 8 in, 2 out]
      }
      event "Decline Button": Value Change {
        # "True: Stop While Loop and Close Dialog"
        n281 = event-data() -> ()  [unwired: 1 in, 1 out]
        n282 = call-poly "Enqueue Message.vi"("Message"="Decline", "Message Queue"=w318) -> ()  [unwired: 8 in, 2 out]
      }
    }
  }
  n283 = timed-loop {
    tunnel: w10 -> [w346]
    shift-right: [w324] -> w6
    shift-left: w9 -> [w343]
    tunnel: [w342] -> w8
    tunnel: w7 -> [w340]
    shift-right: [w338] -> _
    shift-left: w2 -> [w337]
    timing: w5 -> [_]
    timing-out: [_] -> w4
    shift-right: [w336] -> _
    shift-left: w2 -> [w335]
    shift-right: [w334] -> _
    shift-left: _ -> [w333]
    shift-right: [w332] -> _
    shift-left: 0 -> [w331]
    shift-right: [w330] -> _
    shift-left: w2 -> [w329]
    shift-right: [w328] -> _
    shift-left: w2 -> [w327]
    shift-right: [w326] -> _
    shift-left: _ -> [w325]
    tunnel: [w323] -> w1
    stop <- w341 stop-if-true
    n284 = node-c288() -> ()  [unwired: 1 in]
    n285 = call "Dequeue Message.vi"("error in (no error)"=w340, "Message Queue"=w346) -> ("error out"=w339:errorcluster, "Message Data"=w345:variant, "Message"=w344:string, "dup Message Queue"=w323:refnum<queue>)  [unwired: 6 in]
    n286 = case shown="\"Initialize\"" w344 {
      tunnel: w343 -> [w357 w384 w423 w452 w546 w573 w596 w756 w766]
      tunnel: w345 -> [_ _ _ _ _ _ _ _ _]
      tunnel: [w357 w383 w438 w460 w541 w573 w596 w756 w761] -> w324
      tunnel: [w356 w395 w426 w461 w542 w574 w594 w742 w767] -> w342
      tunnel: w339 -> [w356 w395 w439 _ w545 w574 w602 w746 w768]
      tunnel: [_ _ _ _ FALSE FALSE FALSE FALSE TRUE] -> w341
      tunnel: w323 -> [_ _ w440 w464 _ _ w603 w748 _]
      tunnel: [w355 w394 w420 w469 w529 w567 w608 w752 w765] -> w338
      tunnel: w337 -> [w355 w394 _ w469 w529 w567 w608 w752 w765]
      tunnel: [w354 w393 w432 w476 w557 w572 w611 w755 w764] -> w336
      tunnel: w335 -> [w354 w393 w432 w475 w557 w572 w611 w755 w764]
      tunnel: [w353 w392 w433 w472 w556 w571 w610 w754 w763] -> w334
      tunnel: w333 -> [w353 w392 _ w471 w556 w571 w610 w754 w763]
      tunnel: w331 -> [w352 w391 w431 w467 w550 w565 w606 w750 w762]
      tunnel: [w352 w391 w431 w465 w550 w565 w606 w750 w762] -> w332
      tunnel: [w351 w390 w430 w458 w548 w568 w609 w753 w760] -> w330
      tunnel: w329 -> [w351 w390 w430 w457 w548 w568 w609 w753 w760]
      tunnel: [w350 w389 w429 w456 w553 w566 w607 w751 w759] -> w328
      tunnel: w327 -> [w350 w389 w429 w455 w553 w566 w607 w751 w759]
      tunnel: [w349 w388 w428 w454 w549 w564 w605 w749 w758] -> w326
      tunnel: w325 -> [w349 w388 w428 w453 w549 w564 w605 w749 w758]
      frame Default {
      }
      frame "Start Pressed" {
        w382 = T17."Disabled and Grayed Out" ("Disabled")
        # "Close the old connections"
        n287 = Unbundle By Name(w384) -> ("Settings.PID 2 Parameters.Input Device"=w385:T5, "Settings.PID 2 Parameters.Output Device"=w386:T6)
        n288 = Unbundle By Name("Settings Dialog") -> ("Ismatech"=w367:T2, "Masterflex"=w368:T3, "Bronkhorst M13 Flow Meter"=w369:T4, "Setup Parameters"=w370:cluster{"Input Device":T5, "Output Device":T6}, "Bronkhorst M14 Settings"=w373:T13, "Tacmina Settings"=w374:T8, "KNF SIMDOS Settings"=w365:T9, "VICI M50 Settings"=w366:T10, "FLOM Settings"=w376:T11, "SSI PR Settings"=w364:T12, "Calibration Limits.Steps"=w379:dbl, "Calibration Limits"=w380:T24, "File Name"=w381:string)
        n289 = case shown="\"Default\", Default" w386 {
          tunnel: w384 -> [_ w403 w405 w407 _ w410]
          frame "Default", Default {
          }
          frame "Ismatec ISM 831C" {
            n290 = Unbundle By Name(w403) -> ("Settings.Ismatech.VISA resource name"=w404:refnum<visa-resource-name>)
            n291 = VISA Close(VISA resource name=w404) -> ()  [unwired: 1 in, 1 out]
          }
          frame "Masterflex 7550-30" {
            n292 = Unbundle By Name(w405) -> ("Settings.Masterflex.VISA resource name"=w406:refnum<visa-resource-name>)
            n293 = VISA Close(VISA resource name=w406) -> ()  [unwired: 1 in, 1 out]
          }
          frame "VICI" {
            n294 = Unbundle By Name(w407) -> ("Settings.Ismatech.VISA resource name"=w408:refnum<visa-resource-name>)
            n295 = VISA Close(VISA resource name=w408) -> ()  [unwired: 1 in, 1 out]
          }
          frame "Tacmina QI" {
            # "No VISA to Close"
          }
          frame "KNF SIMDOS" {
            n296 = Unbundle By Name(w410) -> ("Settings.KNF SIMDOS Settings.VISA resource name"=w409:refnum<visa-resource-name>)
            n297 = VISA Close(VISA resource name=w409) -> ()  [unwired: 1 in, 1 out]
          }
        }
        n298 = Unbundle(w370) -> ("Input Device"=w371:T5, "Output Device"=w372:T6)
        n299 = case shown="\"KNF SIMDOS\"" w372 {
          tunnel: w365 -> [w400 w401]
          tunnel: [w399 w402] -> w375
          frame "Default", Default {
            n300 = Unbundle(w400) -> ("VISA resource name"=w397:refnum<visa-resource-name>, "Simulated?"=w396:bool)
            n301 = Bundle(cluster=T9 {"VISA resource name"="", "Simulated?"=TRUE} ("KNF Settings"), "VISA resource name"=w397, "Simulated?"=w396) -> (w399:T9)
          }
          frame "KNF SIMDOS" {
            n302 = call "Initialize.vi"("KNF Settings In"=w401) -> ("KNF Settings Out"=w402:T9)  [unwired: 7 in, 3 out]
          }
        }
        n303 = Concatenate Strings(w381, " Calibration Data %Y-%m-%dT%H.%M.%S.csv" ("time format string (%c)")) -> (w362:string)
        n304 = Format Date/Time String(time format string (%c)=w362) -> (date/time string=w360:string)  [unwired: 2 in]
        n305 = Build Path(base path=path "C:/Users/Public/Documents/Calibration Data", name or relative path=w360) -> (appended path=w359:path)
        n306 = Open/Create/Replace File(file path (use dialog)=w359, operation (0:open)=T22."open or create") -> (refnum out=w378:refnum<file>)  [unwired: 4 in, 2 out]
        n307 = case shown="\"Default\", Default" w385 {
          tunnel: w384 -> [_ w412 w413 w415]
          frame "Default", Default {
          }
          frame "Bronkhorst M13" {
            n308 = Unbundle By Name(w412) -> ("Settings.Bronkhorst M13 Flow Meter.VISA resource name"=w411:refnum<visa-resource-name>)
            n309 = VISA Close(VISA resource name=w411) -> ()  [unwired: 1 in, 1 out]
          }
          frame "Bronkhorst M14" {
            n310 = Unbundle By Name(w413) -> ("Settings.Bronkhorst M14.VISA resource name"=w414:refnum<visa-resource-name>)
            n311 = VISA Close(VISA resource name=w414) -> ()  [unwired: 1 in, 1 out]
          }
          frame "Scale Rate of Change" {
            n312 = Unbundle By Name(w415) -> ("Settings.Ismatech.VISA resource name"=w416:refnum<visa-resource-name>)
            n313 = VISA Close(VISA resource name=w416) -> ()  [unwired: 1 in, 1 out]
          }
        }
        n314 = Bundle By Name(cluster=w384, "Settings.Cycle Period"=500.0, "Settings.Ismatech"=w367, "Settings.Masterflex"=w368, "Settings.Bronkhorst M13 Flow Meter"=w369, "Settings.PID 2 Parameters.Input Device"=w371, "Settings.PID 2 Parameters.Output Device"=w372, "Settings.Bronkhorst M14"=w373, "Settings.Tacmina Settings"=w374, "Settings.KNF SIMDOS Settings"=w375, "Settings.VICI M50 Settings"=w366, "Settings.FLOM Settings"=w376, "Settings.SSI PR Settings"=w364, "File Refnum"=w378, "Settings.Calibration Limits.Steps"=w379, "Settings.Calibration Limits"=w380) -> (w383:T1)
        n315 = property on="Cancel Button" class="Bool"("DisabledEnum"=w382) -> ()  [unwired: 2 in, 2 out]
        n316 = property on="Start Button" class="Bool"("DisabledEnum"=w382) -> ()  [unwired: 2 in, 2 out]
      }
      frame "Initialize" {
        n317 = call "Initialize.vi"("error in"=w439, "Pump Calibration Config in"=w423) -> ("error out"=w427:errorcluster, "Pump Calibration Config Out"=w438:T1)  [unwired: 8 in]
        n318 = Unbundle By Name(w423) -> ("Settings.Calibration Limits"=w437:T24)
        n319 = Unbundle By Name(w437) -> ("Minimum (ml/min)"=w421:dbl, "Maximum (ml/min)"=w419:dbl, "Steps"=w418:dbl)
        n320 = Subtract(x=w419, y=w421) -> (x-y=w436:dbl)
        n321 = Subtract(x=w418, y=2.0) -> (x-y=w424:dbl)
        n322 = Decrement(x=w418) -> (x-1=w417:dbl)
        n323 = Divide(x=w436, y=w417) -> (x/y=w434:dbl)
        n324 = for {
          N: w424 -> [_]
          tunnel: w421 -> [w445]
          tunnel: w434 -> [w444]
          tunnel: dbl[] [] -> [w447]
          tunnel: [w446] -> w422 mode=concatenating
          i -> [w443]
          n325 = Increment(x=w443) -> (x+1=w442:i32)
          n326 = Multiply(x=w444, y=w442) -> (x*y=w449:dbl)
          n327 = Add(x=w445, y=w449) -> (x+y=w448:dbl)
          n328 = Build Array (concatenate)(w447, w448) -> (w446:dbl[])
        }
        n329 = Build Array (concatenate)(w421, w422, w419) -> (w420:dbl[])
        "Step Array" <- w420
        n330 = Get Date/Time In Seconds() -> (seconds since 1Jan1904=w433:timestamp)
        n331 = call-poly "Enqueue Message.vi"("error in (no error)"=w427, "Message"="Run", "Message Queue"=w440) -> ("error out"=w426:errorcluster)  [unwired: 7 in, 1 out]
      }
      frame "Run" {
        n332 = Get Date/Time In Seconds() -> (seconds since 1Jan1904=w463:timestamp)
        n333 = Subtract(x=w463, y=w471) -> (x-y=w474:dbl)
        n334 = call "Input.vi"("Pump Calibration Config in"=w452) -> ("error out"=w477:errorcluster, "Pump Calibration Config Out"=w451:T1)  [unwired: 9 in]
        n335 = Greater?(x=w474, y=30.0) -> (0:w470:bool)
        n336 = case shown="True" w470 {
          tunnel: w451 -> [w496 w513]
          tunnel: [w497 w518] -> w476
          tunnel: w475 -> [w498 w518]
          tunnel: [w495 w521] -> w472
          tunnel: w471 -> [w495 _]
          tunnel: w469 -> [w494 w509]
          tunnel: w467 -> [w493 w504]
          tunnel: [w489 w507] -> w466
          tunnel: [w493 w503] -> w465
          tunnel: w464 -> [w492 w514]
          tunnel: w463 -> [w487 _]
          tunnel: [w480 w508] -> w458
          tunnel: w457 -> [w480 w511]
          tunnel: [w479 w505] -> w456
          tunnel: w455 -> [w479 w506]
          tunnel: [w478 w501] -> w454
          tunnel: w453 -> [w478 _]
          frame False {
            w483 = "," ("string")
            n337 = Unbundle By Name(w496) -> ("Flowmeter Output"=w488:dbl, "File Refnum"=w491:refnum<file>)
            n338 = call-poly "Enqueue Message.vi"("Message"="Run", "Message Queue"=w492) -> ()  [unwired: 8 in, 2 out]
            n339 = Index Array(array=w494, index=w493) -> (element=w489:dbl)
            n340 = Number To Fractional String(number=w488) -> (F-format string=w482:string)  [unwired: 3 in]
            n341 = Number To Fractional String(number=w489) -> (F-format string=w484:string)  [unwired: 3 in]
            n342 = Get Date/Time String(seconds (now)=w487) -> (time string=w485:string)  [unwired: 2 in, 1 out]
            n343 = Concatenate Strings(w485, w483, w484, w483, w482, "\r\n") -> (w490:string)
            n344 = Write to Text File(file (use dialog)=w491, text=w490) -> ()  [unwired: 2 in, 3 out]
            n345 = Build Array (concatenate)(w498, w488) -> (w497:dbl[])
          }
          frame True {
            w515 = 15 ("y")
            n346 = Unbundle By Name(w513) -> ("Settings.Calibration Limits.Steps"=w499:dbl)
            n347 = Index Array(array=w509, index=w504) -> (element=w507:dbl)
            n348 = Array Size(array=w518) -> (size(s)=w520:i32)
            n349 = Decrement(x=w499) -> (x-1=w500:dbl)
            n350 = Equal?(x=w504, y=w500) -> (x = y?=w512:bool)
            n351 = Subtract(x=w520, y=w515) -> (x-y=w519:i32)
            n352 = case shown="False" w512 {
              tunnel: w514 -> [w524 w528]
              tunnel: w504 -> [w523 w527]
              tunnel: [w522 w527] -> w503
              frame False {
                n353 = Increment(x=w523) -> (x+1=w522:i32)
                n354 = call-poly "Enqueue Message.vi"("Message"="Run", "Message Queue"=w524) -> ()  [unwired: 8 in, 2 out]
              }
              frame True {
                n355 = call-poly "Enqueue Message.vi"("Message"="Calculate", "Message Queue"=w528) -> ()  [unwired: 8 in, 2 out]
              }
            }
            n356 = Array Subset(array=w518, index=w519) -> (w517:dbl[])  [unwired: 1 in]
            n357 = Add Array Elements(numeric array=w517) -> (sum=w516:dbl)
            n358 = Divide(x=w516, y=w515) -> (x/y=w510:dbl)
            n359 = Build Array (concatenate)(w506, w507) -> (w505:dbl[])
            "X array" <- w505
            n360 = Build Array (concatenate)(w511, w510) -> (w508:dbl[])
            "Y array" <- w508
            n361 = Bundle(w505, w508) -> (w502:cluster{dbl[], dbl[]})  [unwired: 1 in]
            n362 = Build Array(w502) -> (w501:cluster{dbl[], dbl[]}[])
            n363 = local write "Calibration Graph"(w501) -> ()
            n364 = Get Date/Time In Seconds() -> (seconds since 1Jan1904=w521:timestamp)
          }
        }
        n365 = Bundle By Name(cluster=w451, "Speed %"=w466) -> (w468:T1)
        n366 = call "Output.vi"("error in (no error)"=w477, "Pump Calibration Config in"=w468) -> ("error out"=w462:errorcluster, "Pump Calibration Config Out"=w450:T1)  [unwired: 8 in]
        n367 = call "Pump Status.vi"("error in (no error)"=w462, "Pump Calibration Config in"=w450) -> ("error out"=w461:errorcluster, "Pump Calibration Config out"=w460:T1)  [unwired: 8 in]
        n368 = Unbundle By Name(w460) -> ("Pump On?"=→"Pump Status":enum16{"Off", "On", "Not Initialized"})
      }
      frame "Calculate" {
        w534 = "," ("string")
        n369 = call <vilib>:"Linear Fit.vi"("Y"=w548, "X"=w529, "parameter bounds"=T23 {"slope min"=-inf, "slope max"=inf, "intercept min"=-inf, "intercept max"=inf}) -> ("Best Linear Fit"=w547:dbl[], "slope"=w532:dbl, "intercept"=w531:dbl)  [unwired: 8 in, 2 out]
        "Calibration Slope" <- w532
        "Y Intercept" <- w531
        n370 = for {
          tunnel: w529 -> [w562] mode=indexing
          tunnel: w532 -> [w561]
          tunnel: w531 -> [w560]
          tunnel: [w559] -> w530 mode=indexing
          workers-P: _ -> [_]
          n371 = Multiply(x=w562, y=w561) -> (x*y=w563:dbl)
          n372 = Add(x=w563, y=w560) -> (x+y=w559:dbl)
        }
        n373 = call <vilib>:"Goodness of Fit.vi"("Best Fit"=w547, "Y"=w548) -> ("R-square"=w537:dbl)  [unwired: 6 in, 3 out]
        "R^2 Value" <- w537
        n374 = call "Close.vi"("error in (no error)"=w545, "Pump Calibration Config in"=w546) -> ("error out"=w543:errorcluster, "Pump Calibration Config out"=w544:T1)  [unwired: 8 in]
        n375 = Number To Fractional String(number=w532) -> (F-format string=w538:string)  [unwired: 3 in]
        n376 = Number To Fractional String(number=w537) -> (F-format string=w536:string)  [unwired: 3 in]
        n377 = Number To Fractional String(number=w531) -> (F-format string=w533:string)  [unwired: 3 in]
        n378 = call "Pump Status.vi"("error in (no error)"=w543, "Pump Calibration Config in"=w544) -> ("error out"=w542:errorcluster, "Pump Calibration Config out"=w541:T1)  [unwired: 8 in]
        n379 = Concatenate Strings(w534, w534, w534, w538, w534, w536, w534, w533, "\r\n") -> (w539:string)
        n380 = Unbundle By Name(w541) -> ("File Refnum"=w540:refnum<file>)
        n381 = Bundle(w529, w530) -> (w551:cluster{dbl[], dbl[]})  [unwired: 1 in]
        n382 = Bundle(w529, w548) -> (w554:cluster{dbl[], dbl[]})  [unwired: 1 in]
        n383 = Write to Text File(file (use dialog)=w540, text=w539) -> ()  [unwired: 2 in, 3 out]
        n384 = Build Array(w554, w551) -> (→"Calibration Graph":cluster{dbl[], dbl[]}[])
      }
      frame "Close File" {
        n385 = Unbundle By Name(w573) -> ("File Refnum"=w570:refnum<file>)
        n386 = Not A Number/Path/Refnum?(number/path/refnum=w570) -> (NaN/Path/Refnum?=w569:bool)
        n387 = case shown="False" w569 {
          tunnel: w570 -> [w576 _]
          frame False {
            n388 = Close File(refnum=w576) -> ()  [unwired: 1 in, 2 out]
          }
          frame True {
          }
        }
      }
      frame "Accept" {
        w579 = "," ("string")
        w589 = path "C:/Users/Public/Documents/Calibration Data/Pumps Calibration Curves.csv" ("Pump Module Config.Settings.Pump Calibration File")
        n389 = call-poly "Enqueue Message.vi"("error in (no error)"=w602, "Message"="Close File", "Message Queue"=w603) -> ("error out"=w599:errorcluster, "dup Message Queue"=w600:refnum<queue>)  [unwired: 7 in]
        n390 = property on="Calibration Slope" class="DigNum (strict)"() -> ("Value"=w595:dbl)  [unwired: 2 in, 2 out]
        n391 = call-poly "Enqueue Message.vi"("error in (no error)"=w599, "Message"="Exit", "Message Queue"=w600) -> ("error out"=w593:errorcluster)  [unwired: 7 in, 1 out]
        n392 = call-poly <vilib>:"Read Delimited Spreadsheet.vi"("file path (dialog if empty)"=w589, "delimiter (\\t)"="\n" ("delimiter (\\t)")) -> ("all rows"=w583:string[][])  [unwired: 8 in, 5 out]
        n393 = property on="Y Intercept" class="DigNum (strict)"() -> ("Value"=w578:dbl)  [unwired: 2 in, 2 out]
        n394 = property on="File Name" class="Str"(error in=w593) -> (error out=w588:errorcluster, "Text.Text"=w586:string)  [unwired: 1 in, 1 out]
        n395 = Number To Fractional String(number=w595) -> (F-format string=w585:string)  [unwired: 3 in]
        n396 = Number To Fractional String(number=w578) -> (F-format string=w577:string)  [unwired: 3 in]
        n397 = for {
          tunnel: w586 -> [w620]
          tunnel: w583 -> [w619] mode=indexing
          tunnel: [w614] -> w582
          tunnel: [w613] -> w580
          i -> [w613]
          stop <- w614 stop-if-true
          n398 = Index Array(array=w619, index=0) -> (element=w616:string)
          n399 = xnode "Match Regular Expression"("input string"=w616, "regular expression"="^([^,])+") -> ("whole match"=w615:string)  [unwired: 4 in, 4 out]
          n400 = Equal?(x=w615, y=w620) -> (x = y?=w614:bool)
        }
        n401 = Concatenate Strings(w586, w579, w585, w579, w577) -> (w584:string)
        n402 = Open/Create/Replace File(file path (use dialog)=w589, error in=w588, operation (0:open)=T22."replace or create") -> (error out=w587:errorcluster)  [unwired: 3 in, 2 out]
        n403 = Build Array(w584) -> (w581:string[])
        n404 = case shown="False" w582 {
          tunnel: w583 -> [w736 w741]
          tunnel: w580 -> [_ w740]
          tunnel: [w735 w739] -> w591
          tunnel: w581 -> [w737 w738]
          frame False {
            n405 = Build Array (concatenate)(w736, w737) -> (w735:string[][])
          }
          frame True {
            n406 = Replace Array Subset(array=w741, new element=w738, index (row)=w740) -> (w739:string[][])  [unwired: 1 in]
          }
        }
        n407 = call-poly <vilib>:"Write Delimited Spreadsheet.vi"("file path (dialog if empty)"=w589, "2D data"=w591, "append to file? (new file:F)"=TRUE, "error in (no error)"=w587, "delimiter (\\t)"="," ("delimiter (\\t)")) -> ("error out"=w594:errorcluster)  [unwired: 9 in, 1 out]
      }
      frame "Decline" {
        n408 = call-poly "Enqueue Message.vi"("error in (no error)"=w746, "Message"="Close File", "Message Queue"=w748) -> ("error out"=w743:errorcluster, "dup Message Queue"=w744:refnum<queue>)  [unwired: 7 in]
        n409 = call-poly "Enqueue Message.vi"("error in (no error)"=w743, "Message"="Exit", "Message Queue"=w744) -> ("error out"=w742:errorcluster)  [unwired: 7 in, 1 out]
      }
      frame "Exit" {
        n410 = call "Close.vi"("error in (no error)"=w768, "Pump Calibration Config in"=w766) -> ("error out"=w767:errorcluster, "Pump Calibration Config out"=w761:T1)  [unwired: 8 in]
      }
    }
    n411 = node-c288() -> ()  [unwired: 1 in, 1 out]
  }
  "error out" <- w8
  "Pump Calibration Config out" <- w6
  n412 = node-c288(w4) -> ()  [unwired: 1 out]
  n413 = Release Queue(queue=w1) -> ()  [unwired: 2 in, 3 out]
